vi "Marvin.vi"() -> ()   [LabVIEW 2017]
uses:
  Marvin ATP Remake 1.5.18/PCAN_Driver/ControlCAN.llb/CAN Channel.ctl
  Marvin ATP Remake 6.5.18 - Copy/PCAN_Driver/ControlCAN.llb/DevType.ctl
  Marvin ATP Remake 6.5.18/PCAN_Driver/ControlCAN.llb/VCI_INIT_CONFIG.ctl
  Marvin ATP Remake 6.5.18/PCAN_Driver/ControlCAN.llb/InitFlag.ctl
  Marvin ATP Remake 6.5.18/PCAN_Driver/ControlCAN.llb/Fliter.ctl
  Marvin ATP Remake 6.5.18/PCAN_Driver/ControlCAN.llb/Mode.ctl
  <vilib>/Utility/miscctls.llb/LVMinMaxIncTypeDef.ctl
  PCAN_Driver/ControlCAN.llb/VCI_CAN_OBJ.ctl
  PCAN_Driver/ControlCAN.lvlib
panel:
  out "Array 2":dbl[](array[numeric])
  in  "Clear Data Array":bool
  in  "PlayPause Data Array":bool
  out "CAN Data":cluster{"Frame Data":u64, "Frame ID":u32}[](array[cluster]) {"Frame ID" format="%.0x"; "Frame Data" format="%016x"}
  out "Waveform Chart":dbl[](graph)
  in  "Help Button":bool
  in  "Clear Monitor":bool
  out "Array":u64[][](array[numeric]) format="%016x"
  out "Ambient Over temp":bool
  out "Ambient Sensor temp":bool
  out "Ambient Temperature":dbl
  in  "Motor Over Temp":bool
  in  "Speed control":bool
  out "Unit Adress":string
  in  "Serial Send":bool
  in  "Index":u16(ring) items=["1"=1, "2"=2, "3"=3]
  out "read buffer":string
  in  "SetGet":enum16{"Get", "Set"}(ring)
  in  "Function":T1(ring)
  in  "Value":dbl
  in  "Value 1/2":enum16{"1", "2"}(ring)
  out "Msg Count":u32
  in  "Param to Set":u16(ring) items=["EBAY 5F"=95, "AHU 3F"=63, "AHU 2F"=47]
  out "UUT":u8
  out "Horizontal Progress Bar":i32(slide) min=0 max=48 scale=0.0..50.0
  in  "Set Param.":bool
  in  "Serial Monitor":bool caption="Graph Button"
  in  "Serial Com":bool
  in  "VISA resource name":refnum<visa-resource-name>="COM6"
  out "Serial Status":bool
  in  "Graph Button":bool
  in  "Refresh Button":bool
  out "Data Send":u64 format="%016x"
  in  "Motor Speed RPM":u16
  out "Under voltage/Over voltage":bool
  out "Speed error":bool
  out "Derated drive temp":bool
  out "Motor Over temperature":bool
  out "Commutation err":bool
  out "Motor Sensor temp Fauilre":bool
  out "Drive Over temperature":bool
  out "Drive Sensor temp Failure":bool
  out "Motor Phase Current RMS":dbl
  out "ECS State":u16
  out "Motor Speed RPM":dbl
  out "Motor Stator Temp.":dbl
  out "Power transistor Heat sink Temp.":dbl
  out "DC Current":dbl
  out "DC Voltage":dbl
  in  "Can Send":bool
  in  "Stop":bool
  out "Config_CANAT":T8 {"DevType" items=["USB-CAN"=3, "USB-CAN2"=4]; "CanIndex" items=["通道1", "通道2"]; "VCI_INIT_CONFIG"."Fliter" items=["接收所有类型"=3, "只接收标准帧"=4, "只接收扩展帧"=7]; "VCI_INIT_CONFIG"."Mode" items=["正常工作", "自测模式（环回）", "仅侦听模式"]; "VCI_INIT_CONFIG"."InitFlag" items=["使用Flash参数", "使用界面设置参数"]}
  in  "Channel 2":T3 caption="Channel" items=["Channel 1", "Channel 2"]
  out "CAN Status":bool
  out "Driver Version":string
  out "Hall Sensor Fault":bool
  out "Motor Phase Current":dbl
  in  "Motor Phase Current":u16
  # "ver 1.7c"
  # "Marvin"
  # "REDLER TECHNOLOGIES LTD"
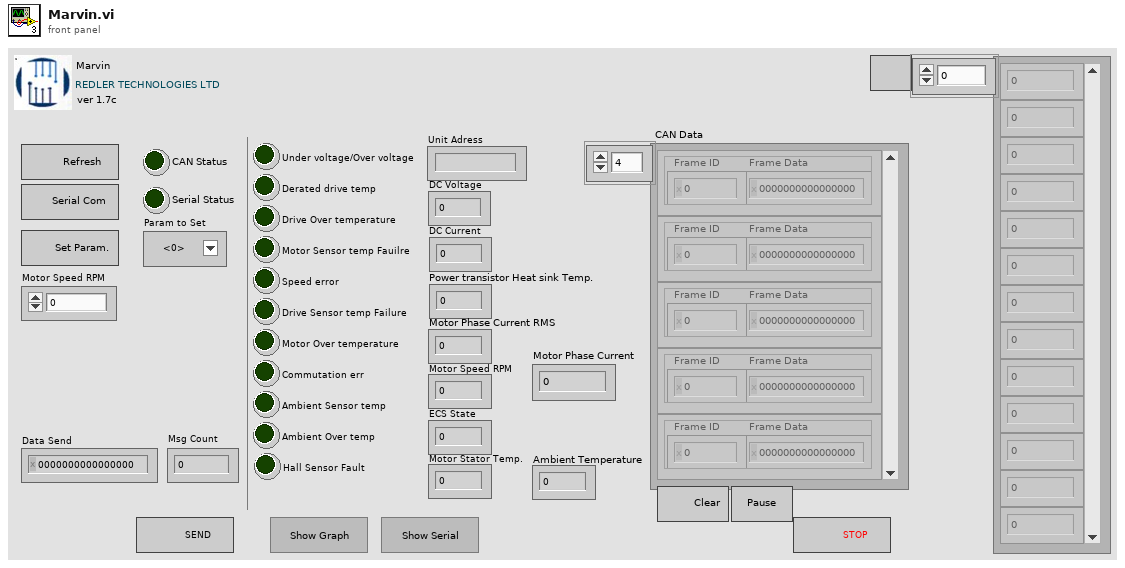
[diagram p1: front panel]
types:
  T1 = enum16{"Enable Conf. EP=1", "Serial Number", "Temperature", "Unit Adress", "Calibration", "Velocity", "Version"}
  T2 = typedef "ControlCAN.lvlib/DevType.ctl" = u32
  T3 = typedef "ControlCAN.lvlib/CAN Channel.ctl" = u32
  T4 = typedef "ControlCAN.lvlib/VCI_INIT_CONFIG.ctl" = cluster{"AccCode":u32, "AccMask":u32, "InitFlag":T5, "Fliter":T6, "Timing0":u8, "Timing1":u8, "Mode":T7}
  T5 = typedef "ControlCAN.lvlib/InitFlag.ctl" = u32
  T6 = typedef "ControlCAN.lvlib/Fliter.ctl" = u8
  T7 = typedef "ControlCAN.lvlib/Mode.ctl" = u8
  T8 = cluster{"DevType":T2, "DevIndex":u32, "CanIndex":T3, "VCI_INIT_CONFIG":T4}
  T9 = cluster{"ID":u32, "MSGTYPE":u8, "LEN":u8, "aDATA":u8[]}[]
  T10 = cluster{"ID":u32, "MSGTYPE":u8, "LEN":u8, "aDATA":u8[]}
  T11 = enum8{"Enabled", "Disabled", "Disabled and Grayed Out"}
  T12 = typedef "LVMinMaxIncTypeDef.ctl" = cluster{"Minimum":dbl, "Maximum":dbl, "Increment":dbl}
  T13 = enum32{"Invalid", "Standard", "Closed", "Hidden", "Minimized", "Maximized"}
  T14 = typedef "ControlCAN.lvlib/VCI_CAN_OBJ.ctl" = cluster{"ID":u32, "TimeStamp":u32, "TimeFlag":u8, "SendType":u8, "RemoteFlag":u8, "ExternFlag":u8, "DataLen":u8, "Data":u8[], "Reserved":u8[]}
  T15 = cluster{"Type":enum16{"接收", "发送"}, "Channel":T3, "Time":timestamp, "VCI_CAN_OBJ":T14}[]
  T16 = cluster{"Type":enum16{"接收", "发送"}, "Channel":T3, "Time":timestamp, "VCI_CAN_OBJ":T14}
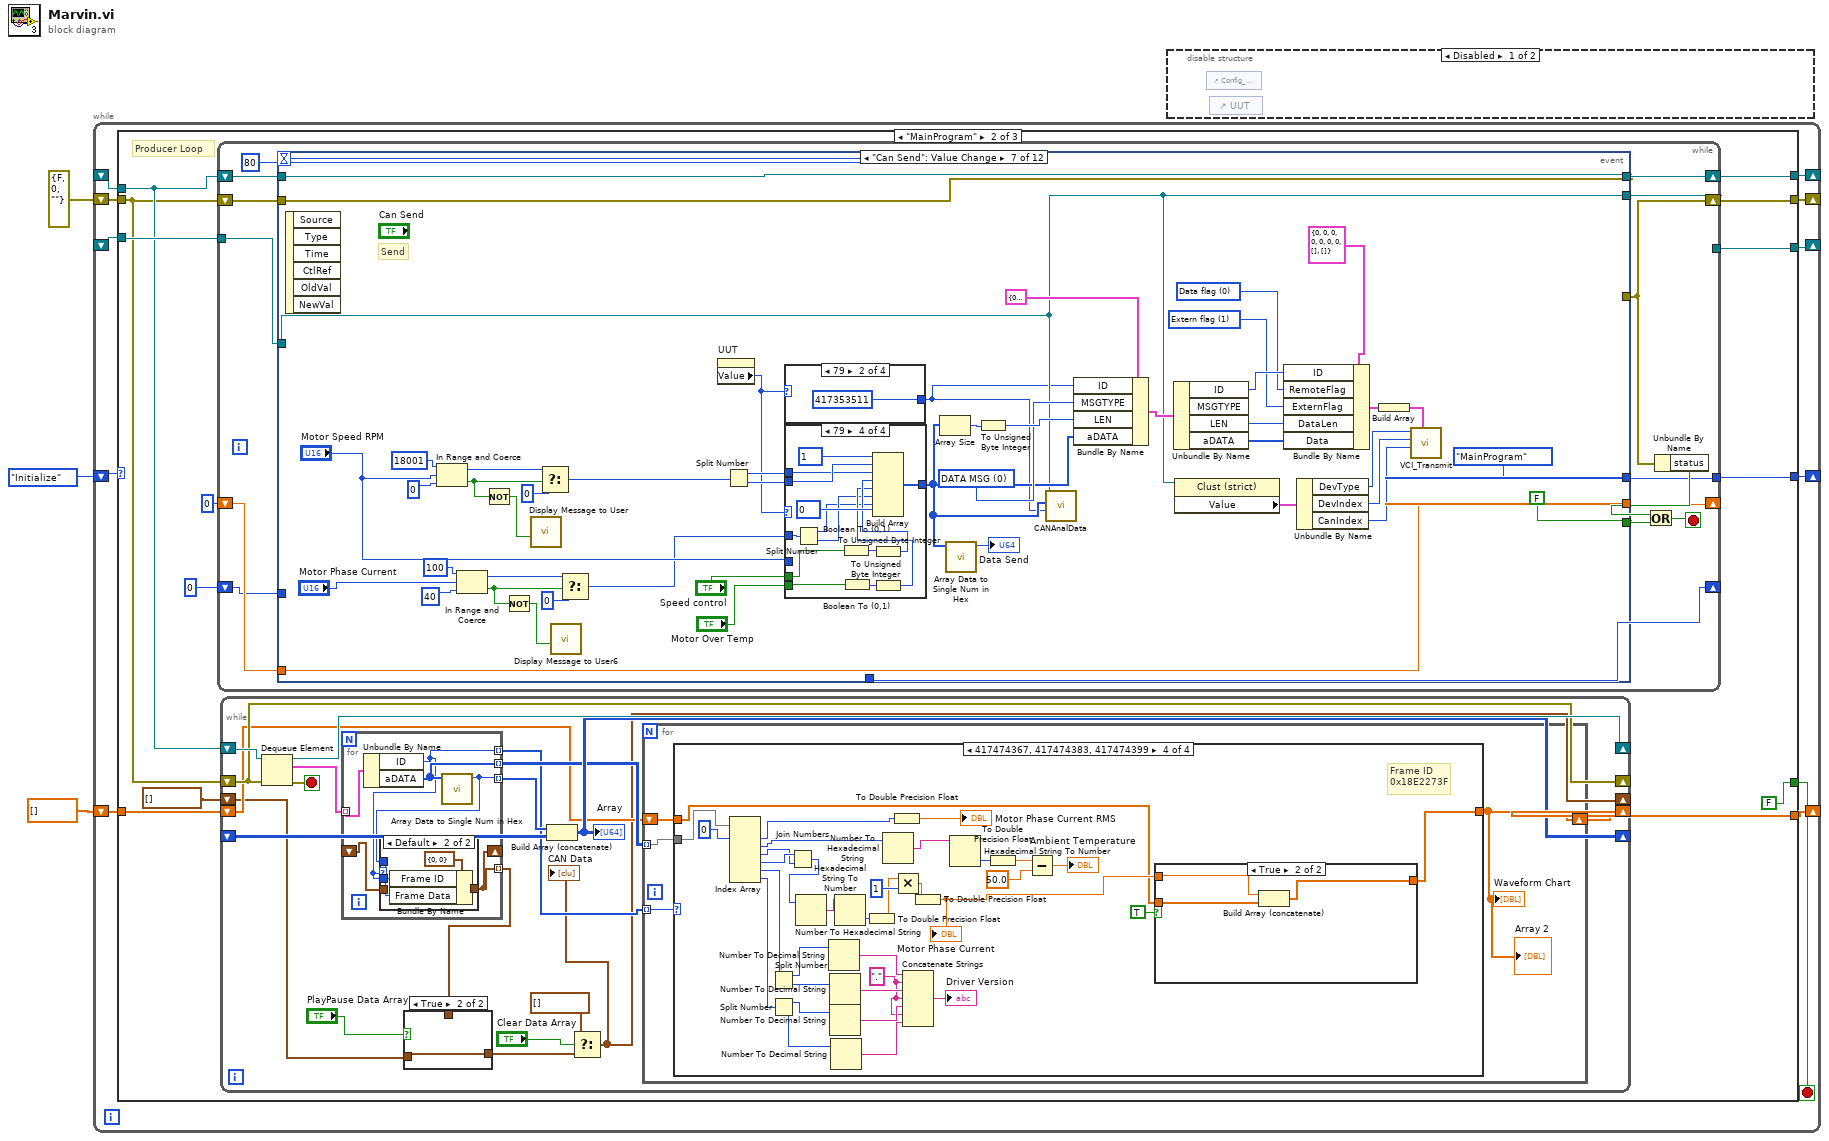
[diagram p0: block diagram]
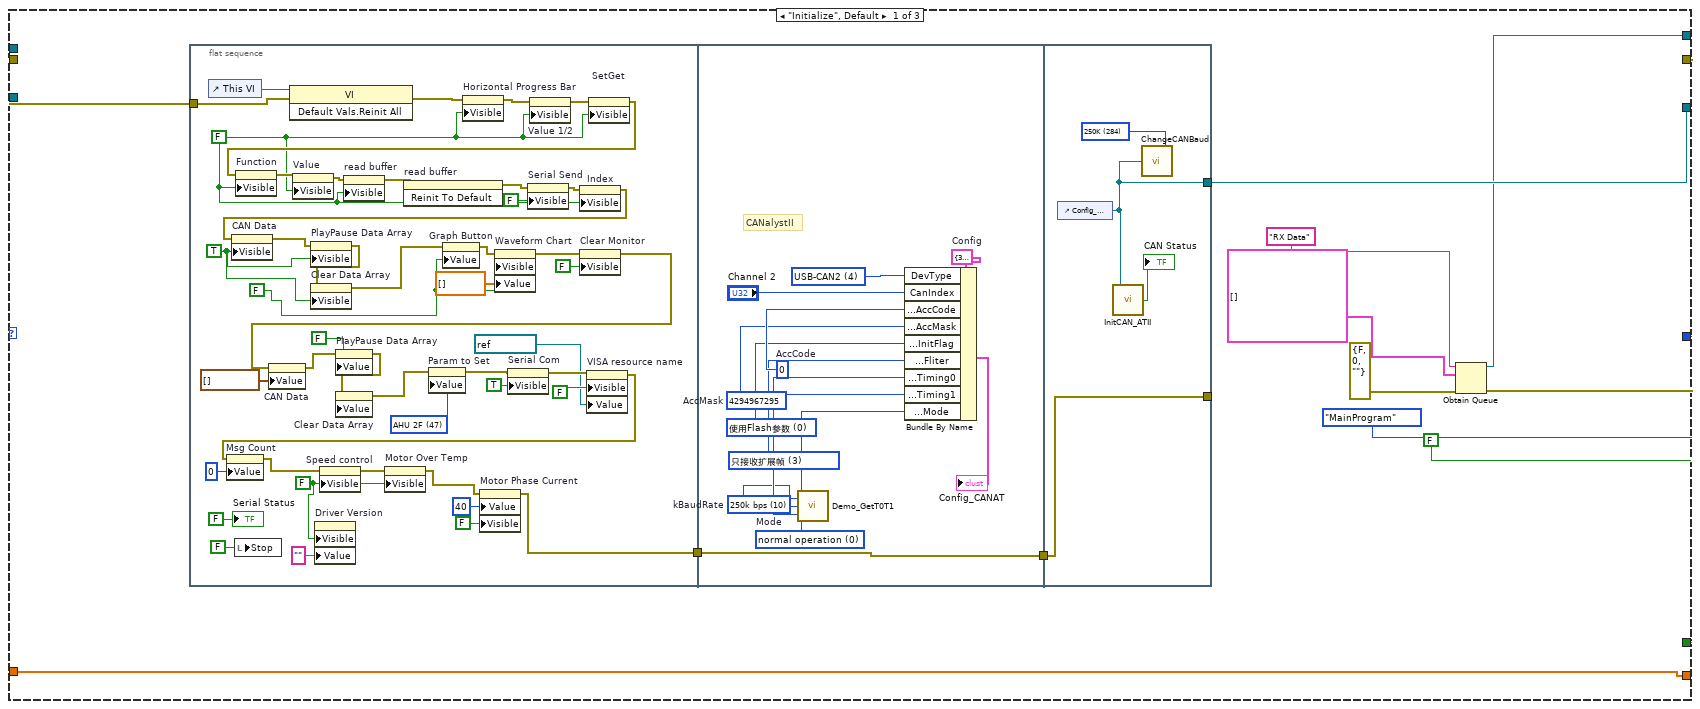
[diagram p3: hidden frame]
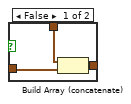
[diagram p4: hidden frame]
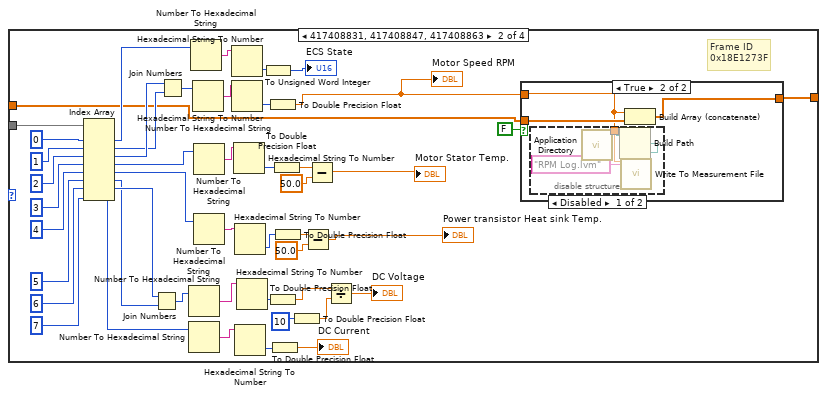
[diagram p6: hidden frame]
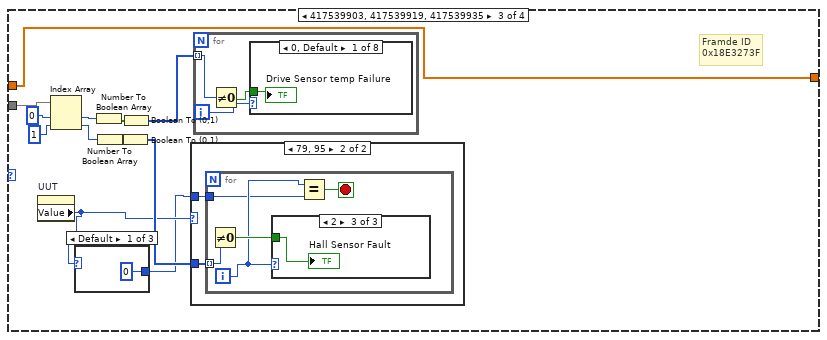
[diagram p9: hidden frame]
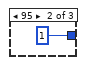
[diagram p10: hidden frame]
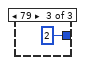
[diagram p11: hidden frame]
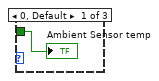
[diagram p13: hidden frame]
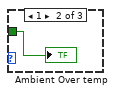
[diagram p14: hidden frame]
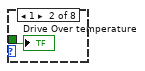
[diagram p15: hidden frame]
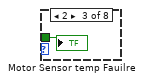
[diagram p16: hidden frame]
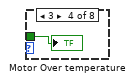
[diagram p17: hidden frame]
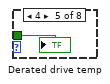
[diagram p18: hidden frame]
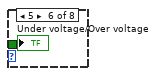
[diagram p19: hidden frame]
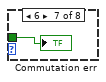
[diagram p20: hidden frame]
diagram:
  n1 = while {
    shift-right: [w9] -> _
    shift-left: enum16{"Stop", "MainProgram", "Initialize"}."Initialize" -> [w14]
    shift-right: [w13] -> _
    shift-left: _ -> [w12]
    shift-right: [w11] -> _
    shift-left: _ -> [w8]
    shift-right: [w10] -> _
    shift-left: errorcluster {"status"=FALSE, "code"=0, "source"=""} ("error out") -> [w7]
    shift-right: [w4] -> _
    shift-left: dbl[] [] -> [w5]
    stop <- w6 stop-if-true
    n2 = case shown="\"MainProgram\"" w14 {
      tunnel: [w26 w100 w1007] -> w13
      tunnel: w12 -> [_ w103 w1007]
      tunnel: [w22 w102 w1008] -> w11
      tunnel: [w21 w101 w1009] -> w10
      tunnel: [enum16{"Stop", "MainProgram", "Initialize"}."MainProgram" w99 enum16{"Stop", "MainProgram", "Initialize"}."Stop"] -> w9
      tunnel: w8 -> [_ w98 w1008]
      tunnel: w7 -> [w19 w97 w1010]
      tunnel: [FALSE ("Stop") FALSE ("Stop") w1006] -> w6
      tunnel: w5 -> [w15 w94 w1004]
      tunnel: [w15 w93 w1004] -> w4
      frame "Initialize", Default {
        n3 = flat-sequence {
          tunnel: w19 -> [w55]
          tunnel: [w29] -> w17
          tunnel: [w74] -> w18
          tunnel: w17 -> [w74]
          tunnel: [w88] -> w26
          tunnel: w18 -> [w87]
          tunnel: [w87] -> _
          frame #0 {
            w38 = FALSE ("PlayPause Data Array")
            w32 = FALSE ("Visible")
            w65 = u16 47 items=["EBAY 5F"=95, "AHU 3F"=63, "AHU 2F"=47] ("Param to Set")
            w33 = TRUE ("Visible")
            w49 = FALSE ("Visible")
            w37 = FALSE ("Graph Button")
            n4 = control-ref of="This VI"() -> (w73:refnum<vi>)
            n5 = local write "Stop"(FALSE ("Stop")) -> ()
            n6 = invoke class="VI" method="Default Vals.Reinit All"(reference=w73, error in=w55) -> (error out=w54:errorcluster)  [unwired: 1 in, 2 out]
            n7 = property on="Driver Version" class="Str"("Visible"=w32, "Value"="" ("Driver Version")) -> ()  [unwired: 2 in, 2 out]
            n8 = property on="Horizontal Progress Bar" class="Slide (strict)"(error in=w54, "Visible"=w49) -> (error out=w63:errorcluster)  [unwired: 1 in, 1 out]
            n9 = property on="Value 1/2" class="Enum (strict)"(error in=w63, "Visible"=w49) -> (error out=w62:errorcluster)  [unwired: 1 in, 1 out]
            n10 = property on="SetGet" class="Enum (strict)"(error in=w62, "Visible"=w49) -> (error out=w61:errorcluster)  [unwired: 1 in, 1 out]
            n11 = property on="Function" class="Enum (strict)"(error in=w61, "Visible"=w49) -> (error out=w60:errorcluster)  [unwired: 1 in, 1 out]
            n12 = property on="Value" class="DigNum (strict)"(error in=w60, "Visible"=w49) -> (error out=w59:errorcluster)  [unwired: 1 in, 1 out]
            n13 = property on="read buffer" class="Str"(error in=w59, "Visible"=w49) -> (error out=w51:errorcluster)  [unwired: 1 in, 1 out]
            n14 = invoke on="read buffer" class="Str" method="Reinit To Default"(error in=w51) -> (error out=w50:errorcluster)  [unwired: 2 in, 2 out]
            n15 = property on="Serial Send" class="Bool (strict)"(error in=w50, "Visible"=FALSE) -> (error out=w58:errorcluster)  [unwired: 1 in, 1 out]
            n16 = property on="Index" class="Ring (strict)"(error in=w58, "Visible"=w49) -> (error out=w44:errorcluster)  [unwired: 1 in, 1 out]
            n17 = property on="CAN Data" class="Arr (strict)"(error in=w44, "Visible"=w33) -> (error out=w36:errorcluster)  [unwired: 1 in, 1 out]
            n18 = property on="PlayPause Data Array" class="Bool (strict)"(error in=w36, "Visible"=w33) -> (error out=w35:errorcluster)  [unwired: 1 in, 1 out]
            n19 = property on="Clear Data Array" class="Bool (strict)"(error in=w35, "Visible"=w33) -> (error out=w34:errorcluster)  [unwired: 1 in, 1 out]
            n20 = property on="Graph Button" class="Bool (strict)"(error in=w34, "Value"=w37) -> (error out=w47:errorcluster)  [unwired: 1 in, 1 out]
            n21 = property on="Waveform Chart" class="WFChart (strict)"(error in=w47, "Visible"=w37, "Value"=dbl[] [] ("Waveform Chart")) -> (error out=w46:errorcluster)  [unwired: 1 in, 1 out]
            n22 = property on="Clear Monitor" class="Bool"(error in=w46, "Visible"=FALSE) -> (error out=w43:errorcluster)  [unwired: 1 in, 1 out]
            n23 = property on="CAN Data" class="Arr (strict)"(error in=w43, "Value"=cluster{"Frame Data":u64, "Frame ID":u32}[] [] ("CAN Data")) -> (error out=w41:errorcluster)  [unwired: 1 in, 1 out]
            n24 = property on="PlayPause Data Array" class="Bool (strict)"(error in=w41, "Value"=w38) -> (error out=w40:errorcluster)  [unwired: 1 in, 1 out]
            n25 = property on="Clear Data Array" class="Bool (strict)"(error in=w40, "Value"=w38) -> (error out=w39:errorcluster)  [unwired: 1 in, 1 out]
            n26 = property on="Param to Set" class="Ring (strict)"(error in=w39, "Value"=w65) -> (error out=w57:errorcluster)  [unwired: 1 in, 1 out]
            n27 = property on="Serial Com" class="Bool"(error in=w57, "Visible"=TRUE) -> (error out=w70:errorcluster)  [unwired: 1 in, 1 out]
            n28 = property on="VISA resource name" class="VISAName"(error in=w70, "Visible"=FALSE, "Value"=refnum<visa-resource-name> "COM1" ("VISA resource name")) -> (error out=w56:errorcluster)  [unwired: 1 in, 1 out]
            n29 = property on="Msg Count" class="DigNum (strict)"(error in=w56, "Value"=u32 0 ("Msg Count")) -> (error out=w53:errorcluster)  [unwired: 1 in, 1 out]
            n30 = property on="Speed control" class="Bool (strict)"(error in=w53, "Visible"=w32) -> (error out=w52:errorcluster)  [unwired: 1 in, 1 out]
            n31 = property on="Motor Over Temp" class="Bool (strict)"(error in=w52, "Visible"=w32) -> (error out=w30:errorcluster)  [unwired: 1 in, 1 out]
            n32 = property on="Motor Phase Current" class="DigNum (strict)"(error in=w30, "Value"=u16 40 ("Motor Phase Current"), "Visible"=FALSE) -> (error out=w29:errorcluster)  [unwired: 1 in, 1 out]
            "Serial Status" <- FALSE ("Serial Status")
          }
          frame #1 {
            w78 = u32 4294967295  # AccMask
            w77 = T5 0 items=["使用Flash参数", "使用界面设置参数"] ("InitFlag")
            w75 = T7 0 items=["normal operation", "Listen-only mode", "test mode"]  # Mode
            w76 = T6 3 items=["接收所有类型"=1, "只接收标准帧"=2, "只接收扩展帧"=3] ("Fliter")
            w82 = u8 10 items=["5k bps"=1, "10k bps"=2, "20k bps"=3, "40k bps"=4, "50k bps"=5, "80k bps"=6, "100k bps"=7, "125k bps"=8, "200k bps"=9, "250k bps"=10, "400k bps"=11, "500k bps"=12, "666k bps"=13, "800k bps"=14, "1000k bps"=15, "33.33k bps"=16, "66.66k bps"=17, "83.33k bps"=18]  # kBaudRate
            w79 = u32 0  # AccCode
            w80 = T2 4 items=["USB-CAN"=3, "USB-CAN2"=4] ("DevType")
            w81 = T8 {"DevType"=3, "DevIndex"=0, "CanIndex"=0, "VCI_INIT_CONFIG"={"AccCode"=0, "AccMask"=0, "InitFlag"=1, "Fliter"=7, "Timing0"=0, "Timing1"=0, "Mode"=0}}  # Config
            # "CANalystII"
            n33 = call "Demo_GetT0T1.vi"("kBaudRate"=w82) -> ("Timing0"=w84:u8, "Timing1"=w85:u8)
            n34 = Bundle By Name(cluster=w81, "DevType"=w80, "CanIndex"="Channel 2", "VCI_INIT_CONFIG.AccCode"=w79, "VCI_INIT_CONFIG.AccMask"=w78, "VCI_INIT_CONFIG.InitFlag"=w77, "VCI_INIT_CONFIG.Fliter"=w76, "VCI_INIT_CONFIG.Timing0"=w84, "VCI_INIT_CONFIG.Timing1"=w85, "VCI_INIT_CONFIG.Mode"=w75) -> (→"Config_CANAT":T8)
          }
          frame #2 {
            w89 = u16 284 items=["1M"=20, "500K"=28, "250K"=284, "125K"=796, "100K"=17199, "50K"=18223, "20K"=21295, "10K"=26415, "5K"=32639] ("baud in")
            n35 = control-ref of="Config_CANAT"() -> (w88:refnum<vi>)
            n36 = call "InitCAN_ATII.vi"("Config"=w88) -> ("Sts"=→"CAN Status":bool)
            n37 = call "ChangeCANBaud.vi"("baud in"=w89, "reference"=w88) -> ()
          }
        }
        n38 = Obtain Queue(name (unnamed)="RX Data", element data type=T9 [], error in (no error)=errorcluster {"status"=FALSE, "code"=0, "source"=""}) -> (queue out=w22:refnum<queue>, error out=w21:errorcluster)  [unwired: 2 in, 1 out]
      }
      frame "MainProgram" {
        # "Producer Loop"
        n39 = while {
          shift-right: [w280] -> w101
          shift-left: w97 -> [w282]
          shift-right: [w281] -> w102
          shift-left: w98 -> [w283]
          tunnel: w103 -> [w284]
          tunnel: [w277] -> w100
          tunnel: [w276] -> w99
          shift-right: [w274] -> _
          shift-left: 0 -> [w275]
          shift-right: [w272] -> _
          shift-left: 0 -> [w273]
          stop <- w285 stop-if-true
          n40 = event shown="[6] \"Can Send\": Value Change" {
            selector: _ -> [_ _ _ _ _ _ _ _ _ _ _ _]
            dyn-events: _ -> [_ _ _ _ _ _ _ _ _ _ _ _]
            timeout: 80 ("Numeric") -> [_ _ _ _ _ _ _ _ _ _ _ _]
            tunnel: w284 -> [w306 w384 w403 w470 w725 w823 w853 w944 w964 w981 w996 w1002]
            tunnel: w283 -> [w303 w385 w406 w471 w724 w824 w874 w945 w963 w982 w993 w999]
            tunnel: w282 -> [w288 w383 w401 w458 w717 w816 w873 w924 w959 w974 w992 w1000]
            tunnel: [w301 w385 w406 w471 w724 w824 w874 w945 w963 w982 w991 w999] -> w281
            tunnel: [w300 w378 w402 w463 w713 w813 w873 w931 w956 w972 w989 w998] -> w280
            tunnel: [FALSE ("Stop") FALSE ("Stop") FALSE ("Stop") FALSE ("Stop") FALSE ("Stop") FALSE ("Stop") FALSE ("Stop") FALSE ("Stop") FALSE ("Stop") FALSE ("Stop") TRUE ("Stop") TRUE ("Stop")] -> w278
            tunnel: [w299 w384 w403 w470 w725 w823 w853 w944 w964 w981 w996 w1002] -> w277
            tunnel: [enum16{"Stop", "MainProgram", "Initialize"}."MainProgram" enum16{"Stop", "MainProgram", "Initialize"}."MainProgram" enum16{"Stop", "MainProgram", "Initialize"}."MainProgram" enum16{"Stop", "MainProgram", "Initialize"}."MainProgram" enum16{"Stop", "MainProgram", "Initialize"}."MainProgram" enum16{"Stop", "MainProgram", "Initialize"}."MainProgram" enum16{"Stop", "MainProgram", "Initialize"}."MainProgram" enum16{"Stop", "MainProgram", "Initialize"}."MainProgram" enum16{"Stop", "MainProgram", "Initialize"}."MainProgram" enum16{"Stop", "MainProgram", "Initialize"}."MainProgram" enum16{"Stop", "MainProgram", "Initialize"}."Stop" enum16{"Stop", "MainProgram", "Initialize"}."Initialize"] -> w276
            tunnel: w275 -> [w295 w388 w399 w459 w715 w827 w839 w940 w955 w970 w988 w997]
            tunnel: [w294 w388 w399 w459 w715 w827 w839 w940 w955 w970 w988 w997] -> w274
            tunnel: w273 -> [w287 _ _ _ _ _ _ _ _ _ _ _]
            tunnel: [w287 _ _ _ _ _ _ _ _ _ _ _] -> w272
            event Timeout {
              n41 = event-data() -> ()  [unwired: 1 in, 3 out]
              n42 = property class="Clust (strict)"(reference=w306) -> (reference out=w299:refnum<vi>, "Value"=w307:T8)  [unwired: 1 in, 1 out]
              n43 = property on="Speed control" class="Bool (strict)"(error in=w288) -> ("Value"=w289:bool)  [unwired: 1 in, 2 out]
              n44 = case shown="True" w289 {
                frame False {
                }
                frame True {
                  n45 = property on="Motor Speed RPM" class="DigNum (strict)"() -> ("Value"=w313:u16)  [unwired: 2 in, 2 out]
                  n46 = control-ref of="Config_CANAT"() -> (w312:refnum<vi>)
                  n47 = control-ref of="UUT"() -> (w311:refnum<vi>)
                  n48 = call "CANSendMotorSpeed.vi"("Remote"=TRUE, "Motor Speed RPM"=w313, "UUT"=w311, "CAN Cluster in"=w312) -> ()  [unwired: 7 in, 1 out]
                }
              }
              n49 = Unbundle By Name(w307) -> ("DevType"=w308:T2, "CanIndex"=w304:T3)
              n50 = property on="Horizontal Progress Bar" class="Slide (strict)"(error in=w288, "Visible"=FALSE) -> (error out=w290:errorcluster)  [unwired: 1 in, 1 out]
              n51 = call "VCI_Receive.vi"("CANIndex"=w304, "DevIndex"=u32 0, "DevType"=w308) -> ("Recieve"=w302:T14[])  [unwired: 3 in, 5 out]
              n52 = Empty Array?(array=w302) -> (empty?=w305:bool)
              n53 = case shown="False" w305 {
                tunnel: w304 -> [w325 _]
                tunnel: w299 -> [w323 _]
                tunnel: w303 -> [w322 w377]
                tunnel: w290 -> [w321 w376]
                tunnel: w302 -> [w326 _]
                tunnel: [w316 w376] -> w300
                tunnel: [w315 w377] -> w301
                tunnel: [w314 0] -> w291
                frame False {
                  n54 = call "Demo_MakeDispBuff.vi"("Channel"=w325, "Type"=enum16{"接收", "发送"}."接收", "OBJs"=w326) -> ("Buffer"=w324:T15)
                  n55 = for {
                    N: 3 -> [_]
                    tunnel: w324 -> [w340]
                    tunnel: w323 -> [w339]
                    tunnel: w322 -> [w330]
                    tunnel: w321 -> [w329]
                    tunnel: [w332] -> w319 mode=indexing
                    tunnel: [w330] -> w318
                    tunnel: [w329] -> w317
                    tunnel: [w328] -> w314
                    i -> [w328]
                    n56 = property class="Clust (strict)"(reference=w339) -> ("Value"=w337:T8)  [unwired: 1 in, 2 out]
                    n57 = Index Array(array=w340, index=w328) -> (element=w333:T16)
                    n58 = Unbundle By Name(w333) -> ("Channel"=w335:T3, "VCI_CAN_OBJ"=w338:T14)  [unwired: 2 out]
                    n59 = Unbundle By Name(w337) -> ("CanIndex"=w336:T3)
                    n60 = Equal?(x=w336, y=w335) -> (x = y?=w334:bool)
                    n61 = case shown="True" w334 {
                      tunnel: w338 -> [_ w356]
                      tunnel: [w341 w352] -> w332
                      tunnel: T10 {"ID"=0, "MSGTYPE"=0, "LEN"=0, "aDATA"=[]} ("Msg") -> [w341 w351]
                      frame False {
                      }
                      frame True {
                        n62 = Unbundle By Name(w356) -> ("ID"=w350:u32, "DataLen"=w355:u8, "Data"=w353:u8[])
                        n63 = Bundle By Name(cluster=w351, "ID"=w350, "MSGTYPE"=u8 0, "LEN"=w355, "aDATA"=w353) -> (w352:T10)
                        n64 = Unbundle By Name(w352) -> ("ID"=w348:u32)
                        n65 = Split Number(x=w348) -> (lo(x)=w349:u16)  [unwired: 1 out]
                        n66 = Split Number(x=w349) -> (lo(x)=w346:u8)  [unwired: 1 out]
                        "UUT" <- w346
                        n67 = case shown="95" w346 {
                          tunnel: ["EBAY 5F" "PUMP 4F" w369 "AHU 3F" "AHU 2F"] -> w345
                          tunnel: [TRUE w366 w370 w371 w373] -> w343
                          tunnel: [TRUE w366 w368 w371 w373] -> w342
                          frame 95 {
                          }
                          frame 79 {
                            w366 = TRUE
                          }
                          frame Default {
                            n68 = property on="Hall Sensor Fault" class="Bool (strict)"() -> ("Visible"=w368:bool)  [unwired: 2 in, 2 out]
                            n69 = property on="Speed control" class="Bool (strict)"() -> ("Visible"=w370:bool)  [unwired: 2 in, 2 out]
                            n70 = property on="Unit Adress" class="Str"() -> ("Value"=w369:string)  [unwired: 2 in, 2 out]
                          }
                          frame 63 {
                            w371 = FALSE
                          }
                          frame 47 {
                            w373 = FALSE
                          }
                        }
                        n71 = Not Equal To 0?(x=w346) -> (x != 0?=w347:bool)
                        n72 = case shown="True" w347 {
                          tunnel: w346 -> [_ w362]
                          tunnel: w345 -> [_ w359]
                          tunnel: [w357 w358] -> w344
                          frame False {
                            n73 = property on="Unit Adress" class="Str"() -> ("Value"=w357:string)  [unwired: 2 in, 2 out]
                          }
                          frame True {
                            n74 = Number To Decimal String(number=w362) -> (decimal integer string=w361:string)  [unwired: 1 in]
                            n75 = call <vilib>:"Space Constant.vi"() -> ("String"=w360:string)
                            n76 = Concatenate Strings(w361, w360, w359) -> (w358:string)
                          }
                        }
                        "Unit Adress" <- w344
                        n77 = property on="Driver Version" class="Str"("Visible"=w343) -> ()  [unwired: 2 in, 2 out]
                        n78 = property on="Hall Sensor Fault" class="Bool (strict)"("Visible"=w342) -> ()  [unwired: 2 in, 2 out]
                        n79 = property on="Motor Phase Current" class="DigNum (strict)"("Visible"=w342) -> ()  [unwired: 2 in, 2 out]
                        n80 = property on="Motor Phase Current" class="DigNum (strict)"("Visible"=w342) -> ()  [unwired: 2 in, 2 out]
                        n81 = property on="Ambient Over temp" class="Bool (strict)"("Visible"=w343) -> ()  [unwired: 2 in, 2 out]
                        n82 = property on="Ambient Sensor temp" class="Bool (strict)"("Visible"=w343) -> ()  [unwired: 2 in, 2 out]
                        n83 = property on="Ambient Temperature" class="DigNum (strict)"("Visible"=w343) -> ()  [unwired: 2 in, 2 out]
                        n84 = property on="Motor Over Temp" class="Bool (strict)"("Visible"=w343) -> ()  [unwired: 2 in, 2 out]
                        n85 = property on="Speed control" class="Bool (strict)"("Visible"=w343) -> ()  [unwired: 2 in, 2 out]
                      }
                    }
                  }
                  n86 = Enqueue Element(queue=w318, element=w319, error in (no error)=w317) -> (queue out=w315:refnum<queue>, error out=w316:errorcluster)  [unwired: 2 out]
                }
                frame True {
                }
              }
              n87 = Divide(x=w291, y=u32 2) -> (x/y=w292:dbl)
              n88 = Add(x=w292, y=w295) -> (x+y=w294:dbl)
              "Msg Count" <- w294
            }
            event "Clear Monitor": Value Change {
              n89 = event-data() -> ()  [unwired: 1 in, 6 out]
              n90 = property on="VISA resource name" class="VISAName"(error in=w383) -> (error out=w382:errorcluster, "Value"=w381:refnum<visa-resource-name>)  [unwired: 1 in, 1 out]
              n91 = disable-structure shown="Enabled" {
                disable-tunnel: w382 -> [w393 w396]
                disable-tunnel: w381 -> [w391 w397]
                disable-tunnel: [w390 ""] -> w380
                disable-tunnel: [w389 w395] -> w379
                frame Disabled {
                  n92 = call "Serial.vi"("error in (no error)"=w393, "Clear Log"=TRUE, "VISA resource name"=w391) -> ("error out"=w389:errorcluster, "read buffer"=w390:string)  [unwired: 7 in]
                }
                frame Enabled {
                  n93 = VISA Flush I/O Buffer(VISA resource name=w397, error in (no error)=w396) -> (error out=w395:errorcluster)  [unwired: 1 in, 1 out]
                }
              }
              n94 = property on="read buffer" class="Str"(error in=w379, "Value"=w380) -> (error out=w378:errorcluster)  [unwired: 1 in, 1 out]
            }
            event "Serial Monitor": Value Change {
              n95 = event-data() -> ()  [unwired: 1 in, 6 out]
              n96 = property on="Serial Status" class="Bool (strict)"(error in=w401) -> (error out=w400:errorcluster, "Value"=w398:bool)  [unwired: 1 in, 1 out]
              n97 = case shown="True" w398 {
                tunnel: w400 -> [w410 w423]
                tunnel: [w408 w428] -> w402
                frame False {
                  n98 = call "Display Message to User3"("error in (no error)"=w410) -> ("error out"=w409:errorcluster)  [unwired: 9 in, 1 out]
                  n99 = property on="Serial Monitor" class="Bool (strict)"(error in=w409, "Value"=FALSE ("Serial Monitor")) -> (error out=w408:errorcluster)  [unwired: 1 in, 1 out]
                }
                frame True {
                  w415 = FALSE ("Visible")
                  w425 = FALSE ("Visible")
                  w426 = u16 1 items=["1"=1, "2"=2, "3"=3] ("Index")
                  n100 = property on="Index" class="Ring (strict)"(error in=w423, "Value"=w426) -> (error out=w422:errorcluster)  [unwired: 1 in, 1 out]
                  n101 = property on="Value 1/2" class="Enum (strict)"(error in=w422, "Visible"=w425) -> (error out=w421:errorcluster)  [unwired: 1 in, 1 out]
                  n102 = property on="Value" class="DigNum (strict)"(error in=w421, "Visible"=w425) -> (error out=w420:errorcluster)  [unwired: 1 in, 1 out]
                  n103 = property on="SetGet" class="Enum (strict)"(error in=w420, "Value"=enum16{"Get", "Set"}."Get" ("SetGet")) -> (error out=w419:errorcluster)  [unwired: 1 in, 1 out]
                  n104 = property on="Serial Send" class="Bool (strict)"(error in=w419, "Visible"=w415) -> (error out=w414:errorcluster)  [unwired: 1 in, 1 out]
                  n105 = property on="Clear Monitor" class="Bool"(error in=w414, "Visible"=w415) -> (error out=w413:errorcluster)  [unwired: 1 in, 1 out]
                  n106 = property on="Function" class="Enum (strict)"(error in=w413, "Value"=T1."Serial Number" ("Function")) -> (error out=w418:errorcluster)  [unwired: 1 in, 1 out]
                  n107 = property on="Index" class="Ring (strict)"(error in=w418, "DisabledEnum"=T11."Disabled and Grayed Out" ("Disabled")) -> (error out=w416:errorcluster)  [unwired: 1 in, 1 out]
                  n108 = case shown="True" "Serial Monitor" {
                    selector: "Serial Monitor" -> [w432 w453]
                    tunnel: w416 -> [w431 w449]
                    tunnel: [w434 w450] -> w428
                    tunnel: [FALSE TRUE] -> w412
                    frame False {
                      n109 = property on="Graph Button" class="Bool (strict)"(error in=w431) -> (error out=w430:errorcluster, "Value"=w429:bool)  [unwired: 1 in, 1 out]
                      n110 = case shown="True" w429 {
                        tunnel: [w438 w443] -> w435
                        tunnel: w430 -> [w440 w446]
                        tunnel: w432 -> [w441 _]
                        frame False {
                          n111 = property on="Waveform Chart" class="WFChart (strict)"(error in=w440, "Visible"=FALSE) -> (error out=w437:errorcluster)  [unwired: 1 in, 1 out]
                          n112 = Not(x=w441) -> (.not. x?=w436:bool)
                          n113 = property on="PlayPause Data Array" class="Bool (strict)"("Visible"=w436) -> ()  [unwired: 2 in, 2 out]
                          n114 = property on="Clear Data Array" class="Bool (strict)"("Visible"=w436) -> ()  [unwired: 2 in, 2 out]
                          n115 = property on="CAN Data" class="Arr (strict)"(error in=w437, "Visible"=w436) -> (error out=w438:errorcluster)  [unwired: 1 in, 1 out]
                        }
                        frame True {
                          w442 = FALSE ("Visible")
                          n116 = property on="Waveform Chart" class="WFChart (strict)"(error in=w446, "Visible"=TRUE) -> (error out=w444:errorcluster)  [unwired: 1 in, 1 out]
                          n117 = property on="PlayPause Data Array" class="Bool (strict)"("Visible"=w442) -> ()  [unwired: 2 in, 2 out]
                          n118 = property on="Clear Data Array" class="Bool (strict)"("Visible"=w442) -> ()  [unwired: 2 in, 2 out]
                          n119 = property on="CAN Data" class="Arr (strict)"(error in=w444, "Visible"=w442) -> (error out=w443:errorcluster)  [unwired: 1 in, 1 out]
                        }
                      }
                      n120 = property on="Serial Monitor" class="Bool (strict)"(error in=w435, "Value"=w432) -> (error out=w434:errorcluster)  [unwired: 1 in, 1 out]
                    }
                    frame True {
                      n121 = Not(x=w453) -> (.not. x?=w447:bool)
                      n122 = property on="PlayPause Data Array" class="Bool (strict)"("Visible"=w447) -> ()  [unwired: 2 in, 2 out]
                      n123 = property on="CAN Data" class="Arr (strict)"(error in=w449, "Visible"=w447) -> (error out=w448:errorcluster)  [unwired: 1 in, 1 out]
                      n124 = property on="Clear Data Array" class="Bool (strict)"("Visible"=w447) -> ()  [unwired: 2 in, 2 out]
                      n125 = property on="Serial Monitor" class="Bool (strict)"(error in=w448, "Value"=w453) -> (error out=w452:errorcluster)  [unwired: 1 in, 1 out]
                      n126 = property on="Graph Button" class="Bool (strict)"(error in=w452, "Value"=w447) -> (error out=w451:errorcluster)  [unwired: 1 in, 1 out]
                      n127 = property on="Waveform Chart" class="WFChart (strict)"(error in=w451, "Visible"=w447) -> (error out=w450:errorcluster)  [unwired: 1 in, 1 out]
                    }
                  }
                  n128 = property on="SetGet" class="Enum (strict)"("Visible"=w412) -> ()  [unwired: 2 in, 2 out]
                  n129 = property on="Index" class="Ring (strict)"("Visible"=w412) -> ()  [unwired: 2 in, 2 out]
                  n130 = property on="Function" class="Enum (strict)"("Visible"=w412) -> ()  [unwired: 2 in, 2 out]
                  n131 = property on="Clear Monitor" class="Bool"("Visible"=w412) -> ()  [unwired: 2 in, 2 out]
                  n132 = property on="Serial Send" class="Bool (strict)"("Visible"=w412) -> ()  [unwired: 2 in, 2 out]
                  n133 = property on="read buffer" class="Str"("Visible"=w412) -> ()  [unwired: 2 in, 2 out]
                }
              }
            }
            event "Serial Send", "Function", "SetGet": Value Change {
              n134 = event-data() -> ()  [unwired: 1 in, 6 out]
              n135 = case shown="\"Enable Conf. EP=1\"" "Function" {
                tunnel: w458 -> [w477 w482 w489 w491 w494 w498 w500 w501]
                tunnel: [w476 w484 w488 w493 w496 w497 w500 w501] -> w456
                frame "Serial Number" {
                  n136 = property on="Index" class="Ring (strict)"(error in=w477, "DisabledEnum"=T11."Disabled and Grayed Out" ("Disabled")) -> (error out=w476:errorcluster)  [unwired: 1 in, 1 out]
                }
                frame "Temperature" {
                  n137 = property on="UUT" class="DigNum (strict)"() -> ("Value"=w479:u8)  [unwired: 2 in, 2 out]
                  n138 = case shown="95" w479 {
                    tunnel: [i32[] [2] ("Disabled Items []") i32[] [3] ("Disabled Items []")] -> w480
                    frame 47, 63, Default {
                    }
                    frame 95 {
                    }
                  }
                  n139 = property on="Index" class="Ring (strict)"(error in=w482, "DisabledEnum"=T11."Enabled" ("Disabled"), "Visible"=TRUE, "Disabled Items []"=w480) -> (error out=w484:errorcluster)  [unwired: 1 in, 1 out]
                }
                frame "Unit Adress" {
                  n140 = property on="Index" class="Ring (strict)"(error in=w489, "DisabledEnum"=T11."Enabled" ("Disabled"), "Visible"=TRUE) -> (error out=w488:errorcluster)  [unwired: 1 in, 1 out]
                }
                frame "Calibration" {
                  n141 = property on="Index" class="Ring (strict)"(error in=w491, "DisabledEnum"=T11."Disabled and Grayed Out" ("Disabled")) -> (error out=w493:errorcluster)  [unwired: 1 in, 1 out]
                }
                frame "Velocity" {
                  n142 = property on="Index" class="Ring (strict)"(error in=w494, "DisabledEnum"=T11."Disabled and Grayed Out" ("Disabled")) -> (error out=w496:errorcluster)  [unwired: 1 in, 1 out]
                }
                frame "Version" {
                  n143 = property on="Index" class="Ring (strict)"(error in=w498, "DisabledEnum"=T11."Disabled and Grayed Out" ("Disabled")) -> (error out=w497:errorcluster)  [unwired: 1 in, 1 out]
                }
                frame "Enable Conf. EP=1" {
                }
                frame Default {
                }
              }
              n144 = property on="VISA resource name" class="VISAName"() -> ("Value"=w472:refnum<visa-resource-name>)  [unwired: 2 in, 2 out]
              n145 = property on="read buffer" class="Str"(error in=w456) -> (error out=w465:errorcluster, "Text.Scroll Position"=w462:u32)  [unwired: 1 in, 1 out]
              n146 = case shown="\"Set\"" "SetGet" {
                tunnel: "Function" -> [w505 w604]
                tunnel: w472 -> [w511 w614]
                tunnel: w465 -> [w508 w603]
                tunnel: "Value" -> [_ w613]
                tunnel: "Value 1/2" -> [_ w611]
                tunnel: "Index" -> [w506 w608]
                tunnel: [w510 w606] -> w464
                tunnel: [w503 w605] -> w469
                tunnel: "Serial Send" -> [w502 w595]
                frame "Get", Default {
                  w509 = FALSE ("Visible")
                  n147 = property on="Value" class="DigNum (strict)"(error in=w508, "Visible"=w509) -> (error out=w507:errorcluster)  [unwired: 1 in, 1 out]
                  n148 = property on="Value 1/2" class="Enum (strict)"(error in=w507, "Visible"=w509) -> (error out=w504:errorcluster)  [unwired: 1 in, 1 out]
                  n149 = case shown="True" w502 {
                    tunnel: w511 -> [_ w522]
                    tunnel: [w512 w517] -> w510
                    tunnel: w506 -> [_ w521]
                    tunnel: w505 -> [_ w520]
                    tunnel: w504 -> [w512 w519]
                    tunnel: [w513 w515] -> w503
                    frame False {
                      n150 = property on="read buffer" class="Str"() -> ("Value"=w513:string)  [unwired: 2 in, 2 out]
                    }
                    frame True {
                      n151 = case shown="\"Serial Number\"" w520 {
                        tunnel: w522 -> [w527 w545 w561 w570 w577 w588 _]
                        tunnel: w519 -> [w525 w536 w551 w565 w575 w586 w593]
                        tunnel: [w530 w546 w562 w571 w581 w589 w593] -> w517
                        tunnel: [w529 w547 w560 w572 w582 w584 "Cannot perform operation.\n" ("read buffer")] -> w516
                        tunnel: w521 -> [_ w540 w553 _ _ _ _]
                        frame "Serial Number" {
                          n152 = property on="Index" class="Ring (strict)"(error in=w525, "DisabledEnum"=T11."Disabled and Grayed Out" ("Disabled")) -> (error out=w524:errorcluster)  [unwired: 1 in, 1 out]
                          n153 = Concatenate Strings("SN" ("string"), "\r\n" ("write buffer")) -> (w528:string)
                          n154 = call "Serial.vi"("error in (no error)"=w524, "Clear Log"=FALSE, "write buffer"=w528, "VISA resource name"=w527) -> ("error out"=w530:errorcluster, "read buffer"=w529:string)  [unwired: 6 in]
                        }
                        frame "Temperature" {
                          n155 = Number To Decimal String(number=w540) -> (decimal integer string=w539:string)  [unwired: 1 in]
                          n156 = property on="Index" class="Ring (strict)"(error in=w536, "DisabledEnum"=T11."Enabled" ("Disabled"), "Visible"=TRUE) -> (error out=w535:errorcluster)  [unwired: 1 in, 1 out]
                          n157 = Concatenate Strings("TA" ("string"), "[", w539, "]", "\r\n" ("write buffer")) -> (w541:string)
                          n158 = call "Serial.vi"("error in (no error)"=w535, "Clear Log"=FALSE, "write buffer"=w541, "VISA resource name"=w545) -> ("error out"=w546:errorcluster, "read buffer"=w547:string)  [unwired: 6 in]
                        }
                        frame "Unit Adress" {
                          n159 = Number To Decimal String(number=w553) -> (decimal integer string=w559:string)  [unwired: 1 in]
                          n160 = property on="Index" class="Ring (strict)"(error in=w551, "DisabledEnum"=T11."Enabled" ("Disabled"), "Visible"=TRUE) -> (error out=w550:errorcluster)  [unwired: 1 in, 1 out]
                          n161 = Concatenate Strings("UA" ("string"), "[", w559, "]", "\r\n" ("write buffer")) -> (w554:string)
                          n162 = call "Serial.vi"("error in (no error)"=w550, "Clear Log"=FALSE, "write buffer"=w554, "VISA resource name"=w561) -> ("error out"=w562:errorcluster, "read buffer"=w560:string)  [unwired: 6 in]
                        }
                        frame "Calibration" {
                          n163 = property on="Index" class="Ring (strict)"(error in=w565, "DisabledEnum"=T11."Disabled and Grayed Out" ("Disabled")) -> (error out=w564:errorcluster)  [unwired: 1 in, 1 out]
                          n164 = Concatenate Strings("CC" ("string"), "\r\n" ("write buffer")) -> (w568:string)
                          n165 = call "Serial.vi"("error in (no error)"=w564, "Clear Log"=FALSE, "write buffer"=w568, "VISA resource name"=w570) -> ("error out"=w571:errorcluster, "read buffer"=w572:string)  [unwired: 6 in]
                        }
                        frame "Velocity" {
                          n166 = property on="Index" class="Ring (strict)"(error in=w575, "DisabledEnum"=T11."Disabled and Grayed Out" ("Disabled")) -> (error out=w574:errorcluster)  [unwired: 1 in, 1 out]
                          n167 = Concatenate Strings("VC" ("string"), "\r\n" ("write buffer")) -> (w578:string)
                          n168 = call "Serial.vi"("error in (no error)"=w574, "Clear Log"=FALSE, "write buffer"=w578, "VISA resource name"=w577) -> ("error out"=w581:errorcluster, "read buffer"=w582:string)  [unwired: 6 in]
                        }
                        frame "Version" {
                          n169 = Concatenate Strings("VR" ("string"), "\r\n" ("write buffer")) -> (w590:string)
                          n170 = property on="Index" class="Ring (strict)"(error in=w586, "DisabledEnum"=T11."Disabled and Grayed Out" ("Disabled")) -> (error out=w585:errorcluster)  [unwired: 1 in, 1 out]
                          n171 = call "Serial.vi"("error in (no error)"=w585, "Clear Log"=FALSE, "write buffer"=w590, "VISA resource name"=w588) -> ("error out"=w589:errorcluster, "read buffer"=w584:string)  [unwired: 6 in]
                        }
                        frame Default {
                        }
                      }
                      n172 = property on="Serial Send" class="Bool (strict)"(error in=w517, "Value"=FALSE ("Serial Send")) -> ()  [unwired: 1 in, 2 out]
                      n173 = property on="read buffer" class="Str"() -> ("Value"=w514:string)  [unwired: 2 in, 2 out]
                      n174 = Concatenate Strings(w514, w516) -> (w515:string)
                    }
                  }
                }
                frame "Set" {
                  n175 = To Unsigned Long Integer(number=w613) -> (unsigned 32bit integer=w609:u32)
                  n176 = Number To Decimal String(number=w608) -> (decimal integer string=w607:string)  [unwired: 1 in]
                  n177 = Number To Decimal String(number=w611) -> (decimal integer string=w610:string)  [unwired: 1 in]
                  n178 = case shown="Default" w604 {
                    tunnel: w603 -> [w688 w692 w696 w700 w704 w708 w710 w712]
                    tunnel: [FALSE TRUE TRUE FALSE FALSE FALSE w709 w711] -> w601
                    tunnel: [TRUE TRUE TRUE FALSE TRUE FALSE w709 w711] -> w600
                    tunnel: [FALSE FALSE FALSE TRUE FALSE FALSE w709 w711] -> w599
                    tunnel: [w688 w692 w696 w700 w704 w708 w710 w712] -> w597
                    frame "Serial Number" {
                    }
                    frame "Temperature" {
                    }
                    frame "Unit Adress" {
                    }
                    frame "Calibration" {
                    }
                    frame "Velocity" {
                    }
                    frame "Version" {
                    }
                    frame "Enable Conf. EP=1" {
                      w709 = FALSE
                    }
                    frame Default {
                      w711 = FALSE
                    }
                  }
                  n179 = Number To Decimal String(number=w609) -> (decimal integer string=w612:string)  [unwired: 1 in]
                  n180 = property on="Index" class="Ring (strict)"(error in=w597, "Visible"=w601) -> (error out=w602:errorcluster)  [unwired: 1 in, 1 out]
                  n181 = property on="Value" class="DigNum (strict)"(error in=w602, "Visible"=w600) -> (error out=w598:errorcluster)  [unwired: 1 in, 1 out]
                  n182 = property on="Value 1/2" class="Enum (strict)"(error in=w598, "Visible"=w599) -> (error out=w596:errorcluster)  [unwired: 1 in, 1 out]
                  n183 = case shown="True" w595 {
                    tunnel: w614 -> [_ w628]
                    tunnel: w612 -> [_ w627]
                    tunnel: w610 -> [_ w626]
                    tunnel: w609 -> [_ w625]
                    tunnel: w607 -> [_ w624]
                    tunnel: [w615 w623] -> w606
                    tunnel: [w616 w622] -> w605
                    tunnel: w604 -> [_ w620]
                    tunnel: w596 -> [w615 w619]
                    frame False {
                      n184 = property on="read buffer" class="Str"() -> ("Value"=w616:string)  [unwired: 2 in, 2 out]
                    }
                    frame True {
                      n185 = flat-sequence {
                        tunnel: [w632] -> w630
                        tunnel: w619 -> [w632]
                        frame #0 {
                          n186 = Wait (ms)(milliseconds to wait=u32 50) -> ()  [unwired: 1 out]
                        }
                      }
                      n187 = case shown="\"Velocity\"" w620 {
                        tunnel: [w635 w641 w650 w658 w676 "EP=1\r\n" ("write buffer") "Cannot perform operation.\n" ("read buffer")] -> w621
                        tunnel: w630 -> [w634 w640 w649 w663 w667 w679 w681]
                        tunnel: [w634 w640 w649 w663 w664 w679 w681] -> w629
                        tunnel: w627 -> [w636 w642 w655 _ _ _ _]
                        tunnel: w626 -> [_ _ _ w659 _ _ _]
                        tunnel: w625 -> [_ _ _ _ w668 _ _]
                        tunnel: w624 -> [_ w643 w653 _ _ _ _]
                        frame "Serial Number" {
                          n188 = Concatenate Strings("SN" ("write buffer"), "=" ("string"), w636, "\r\n" ("write buffer")) -> (w635:string)
                        }
                        frame "Temperature" {
                          n189 = Concatenate Strings("TA" ("string"), "[", w643, "]", "=" ("string"), w642, "\r\n" ("write buffer")) -> (w641:string)
                        }
                        frame "Unit Adress" {
                          n190 = Concatenate Strings("UA" ("string"), "[", w653, "]", "=" ("string"), w655, "\r\n" ("write buffer")) -> (w650:string)
                        }
                        frame "Calibration" {
                          n191 = Concatenate Strings("CC" ("string"), "=" ("string"), w659, "\r\n" ("write buffer")) -> (w658:string)
                        }
                        frame "Velocity" {
                          n192 = In Range and Coerce(upper limit=u16 18001, x=w668, lower limit=u16 0) -> (coerced(x)=w674:u32, In Range?=w672:bool)
                          n193 = Not(x=w672) -> (.not. x?=w673:bool)
                          n194 = Select(t=w674, s=w672, f=u16 0) -> (s? t:f=w666:u32)
                          n195 = Number To Decimal String(number=w666) -> (decimal integer string=w665:string)  [unwired: 1 in]
                          n196 = Concatenate Strings("VC" ("write buffer"), "=" ("string"), w665, "\r\n" ("write buffer")) -> (w676:string)
                          n197 = call "Display Message to User2"("error in (no error)"=w667, "Enable"=w673) -> ("error out"=w664:errorcluster)  [unwired: 8 in, 1 out]
                        }
                        frame "Enable Conf. EP=1" {
                        }
                        frame Default {
                        }
                      }
                      n198 = property on="read buffer" class="Str"() -> ("Value"=w617:string)  [unwired: 2 in, 2 out]
                      n199 = VISA Write(VISA resource name=w628, write buffer=w621, error in (no error)=w629) -> (error out=w631:errorcluster)  [unwired: 2 out]
                      n200 = Concatenate Strings(w617, w621) -> (w622:string)
                      n201 = property on="Serial Send" class="Bool (strict)"("Value"=FALSE ("Serial Send")) -> ()  [unwired: 2 in, 2 out]
                      n202 = flat-sequence {
                        tunnel: w631 -> [w683]
                        tunnel: [w683] -> w623
                        frame #0 {
                          n203 = Wait (ms)(milliseconds to wait=u32 50) -> ()  [unwired: 1 out]
                        }
                      }
                    }
                  }
                }
              }
              "read buffer" <- w469
              n204 = Add(x=u32 5, y=w462) -> (x+y=w461:u32)
              n205 = property on="read buffer" class="Str"(error in=w464, "Text.Scroll Position"=w461) -> (error out=w463:errorcluster)  [unwired: 1 in, 1 out]
            }
            event "Set Param.": Value Change {
              n206 = event-data() -> ()  [unwired: 1 in, 6 out]
              n207 = property on="Serial Status" class="Bool (strict)"(error in=w717) -> (error out=w716:errorcluster, "Value"=w721:bool)  [unwired: 1 in, 1 out]
              n208 = case shown="True" w721 {
                tunnel: w716 -> [w733 w746]
                tunnel: [w732 w742] -> w719
                frame False {
                  n209 = call "Display Message to User4"("error in (no error)"=w733) -> ("error out"=w732:errorcluster)  [unwired: 9 in, 1 out]
                }
                frame True {
                  w735 = FALSE ("Visible")
                  n210 = property on="Speed control" class="Bool (strict)"(error in=w746, "Visible"=FALSE) -> (error out=w745:errorcluster)  [unwired: 1 in, 1 out]
                  n211 = case shown="47" "Param to Set" {
                    tunnel: [w799 w803 w807] -> w761
                    tunnel: w745 -> [w798 w802 w806]
                    tunnel: [w798 w802 w806] -> w749
                    frame 95, Default {
                      n212 = call <vilib>:"Application Directory.vi"() -> ("Application Directory"=w801:path)
                      n213 = Build Path(base path=w801, name or relative path="data\\Marvin_EBAY_params_RRPAR000017_95_v0.2.txt") -> (appended path=w799:path)
                    }
                    frame 63 {
                      n214 = call <vilib>:"Application Directory.vi"() -> ("Application Directory"=w805:path)
                      n215 = Build Path(base path=w805, name or relative path="data\\Marvin_AHU_params_RRPAR000016_63_v0.2.txt") -> (appended path=w803:path)
                    }
                    frame 47 {
                      n216 = call <vilib>:"Application Directory.vi"() -> ("Application Directory"=w809:path)
                      n217 = Build Path(base path=w809, name or relative path="data\\Marvin_AHU_params_RRPAR000015_47_v0.2.txt") -> (appended path=w807:path)
                    }
                  }
                  n218 = property on="read buffer" class="Str"(error in=w749, "Visible"=TRUE) -> (error out=w737:errorcluster)  [unwired: 1 in, 1 out]
                  n219 = property on="CAN Data" class="Arr (strict)"(error in=w737, "Visible"=w735) -> (error out=w736:errorcluster)  [unwired: 1 in, 1 out]
                  n220 = property on="PlayPause Data Array" class="Bool (strict)"("Visible"=w735) -> ()  [unwired: 2 in, 2 out]
                  n221 = property on="Clear Data Array" class="Bool (strict)"("Visible"=w735) -> ()  [unwired: 2 in, 2 out]
                  n222 = property on="Horizontal Progress Bar" class="Slide (strict)"(error in=w736, "Visible"=TRUE, "Value"=u8 0 ("Horizontal Progress Bar")) -> (error out=w744:errorcluster)  [unwired: 1 in, 1 out]
                  n223 = call <vilib>:"Read Characters From File.vi"("file path (dialog if empty)"=w761) -> ("character string"=w762:string)  [unwired: 5 in, 3 out]
                  n224 = while {
                    shift-right: [w790] -> _
                    shift-left: w762 -> [w791]
                    shift-right: [w786] -> w747
                    shift-left: string[] [] -> [w787]
                    tunnel: w744 -> [w779]
                    tunnel: [w779] -> w759
                    stop <- w792 stop-if-true
                    n225 = Match Pattern(string=w791, regular expression="\r\n") -> (before substring=w788:string, after substring=w790:string, offset past match=w789:i32)  [unwired: 1 in, 1 out]
                    n226 = call <vilib>:"Trim Whitespace.vi"("string"=w788) -> ("trimmed string"=w785:string)  [unwired: 1 in]
                    n227 = Equal?(x=w789, y=-1) -> (x = y?=w792:bool)
                    n228 = To Upper Case(1:w785) -> (0:w783:string)
                    n229 = String Length(string=w783) -> (length=w782:i32)
                    n230 = Greater?(x=w782, y=3) -> (0:w780:bool)
                    n231 = case shown="True" w780 {
                      tunnel: w787 -> [w794 w797]
                      tunnel: [w794 w796] -> w786
                      tunnel: w783 -> [_ w795]
                      frame False {
                      }
                      frame True {
                        n232 = Build Array (concatenate)(w797, w795) -> (w796:string[])
                      }
                    }
                  }
                  n233 = property on="VISA resource name" class="VISAName"(error in=w759) -> (error out=w752:errorcluster, "Value"=w741:refnum<visa-resource-name>)  [unwired: 1 in, 1 out]
                  n234 = Build Array (concatenate)(w747, string[] ["MT", "VR", "SN"] ("array")) -> (w756:string[])
                  n235 = Array Size(array=w756) -> (size(s)=w748:i32)
                  n236 = Bundle By Name(cluster=T12 {"Minimum"=0.0, "Maximum"=0.0, "Increment"=0.0} ("Data Entry Limits"), "Minimum"=0.0, "Maximum"=w748) -> (w754:T12)
                  n237 = property on="Horizontal Progress Bar" class="Slide (strict)"(error in=w752, "Data Range"=w754) -> (error out=w740:errorcluster)  [unwired: 1 in, 1 out]
                  n238 = property on="read buffer" class="Str"(error in=w740) -> (error out=w739:errorcluster, "Text.Scroll Position"=w738:u32)  [unwired: 1 in, 1 out]
                  n239 = for {
                    tunnel: w756 -> [w770] mode=indexing
                    tunnel: w741 -> [w776]
                    tunnel: w739 -> [w775]
                    tunnel: [w767] -> w743
                    tunnel: w738 -> [w766]
                    i -> [w765]
                    n240 = Concatenate Strings(w770, "\r\n" ("string")) -> (w768:string)
                    n241 = VISA Write(VISA resource name=w776, write buffer=w768, error in (no error)=w775) -> (error out=w774:errorcluster)  [unwired: 2 out]
                    n242 = flat-sequence {
                      tunnel: w774 -> [w777]
                      tunnel: [w777] -> w767
                      frame #0 {
                        n243 = Wait (ms)(milliseconds to wait=u32 50) -> ()  [unwired: 1 out]
                      }
                    }
                    n244 = Add(x=w766, y=w765) -> (x+y=w764:u32)
                    n245 = feedback #1("") -> (w772:string)
                    n246 = Concatenate Strings(w772, w768) -> (w773:string)
                    n247 = feedback-in #1(w773) -> ()
                    n248 = property on="read buffer" class="Str"("Value"=w773, "Text.Scroll Position"=w764) -> ()  [unwired: 2 in, 2 out]
                    "Horizontal Progress Bar" <- w765
                  }
                  n249 = VISA Flush I/O Buffer(VISA resource name=w741, error in (no error)=w743) -> (error out=w742:errorcluster)  [unwired: 1 in, 1 out]
                }
              }
              n250 = property on="Serial Monitor" class="Bool (strict)"(error in=w719) -> (error out=w718:errorcluster, "Value"=w720:bool)  [unwired: 1 in, 1 out]
              n251 = case shown="False" w720 {
                tunnel: w718 -> [w730 w731]
                tunnel: [w727 w731] -> w714
                frame False {
                  w726 = TRUE ("Visible")
                  n252 = property on="PlayPause Data Array" class="Bool (strict)"("Visible"=w726) -> ()  [unwired: 2 in, 2 out]
                  n253 = property on="read buffer" class="Str"(error in=w730, "Visible"=FALSE) -> (error out=w728:errorcluster)  [unwired: 1 in, 1 out]
                  n254 = property on="Clear Data Array" class="Bool (strict)"("Visible"=w726) -> ()  [unwired: 2 in, 2 out]
                  n255 = property on="CAN Data" class="Arr (strict)"(error in=w728, "Visible"=w726) -> (error out=w727:errorcluster)  [unwired: 1 in, 1 out]
                }
                frame True {
                }
              }
              n256 = call "Display Message to User5"("error in (no error)"=w714) -> ("error out"=w713:errorcluster)  [unwired: 9 in, 1 out]
            }
            event "Help Button": Value Change {
              n257 = event-data() -> ()  [unwired: 1 in, 6 out]
              n258 = control-ref of="This VI"() -> (w818:refnum<vi>)
              n259 = property class="VI"(reference=w818, error in=w816, "FP:Transparency"=u8 25 ("Front Panel Window:Transparency")) -> (reference out=w812:refnum<vi>, error out=w815:errorcluster)
              n260 = vi-ref "Help.vi"() -> (w822:refnum<vi>)
              n261 = invoke class="VI" method="FP.Open"(reference=w822, error in=w815, "Activate"=TRUE ("Activate?"), "State"=T13."Standard") -> (error out=w821:errorcluster)  [unwired: 1 in, 4 out]
              n262 = call "Help.vi"("error in"=w821, "TesterSWVersion"="1.7") -> ("error out"=w814:errorcluster)  [unwired: 6 in]
              n263 = property class="VI"(reference=w812, error in=w814, "FP:Transparency"=u8 0 ("Front Panel Window:Transparency")) -> (error out=w813:errorcluster)  [unwired: 1 out]
            }
            event "Can Send": Value Change {
              w857 = u8 0 items=["STATUS"=128, "EXTENDED"=2, "RTR"=1, "DATA MSG"=0] ("MSGTYPE")
              w862 = u8 1 items=["Standart flag", "Extern flag"] ("Format")
              w861 = u8 0 items=["Data flag", "Remote flag"] ("Type")
              # "Send"
              n264 = event-data() -> ()  [unwired: 1 in, 6 out]
              n265 = In Range and Coerce(upper limit=u16 18001, x="Motor Speed RPM", lower limit=u16 0) -> (coerced(x)=w844:u16, In Range?=w842:bool)
              n266 = In Range and Coerce(upper limit=u16 100, x="Motor Phase Current", lower limit=u16 40) -> (coerced(x)=w833:u16, In Range?=w835:bool)
              n267 = Not(x=w842) -> (.not. x?=w843:bool)
              n268 = Not(x=w835) -> (.not. x?=w834:bool)
              n269 = call "Display Message to User"("Enable"=w843) -> ()  [unwired: 9 in, 2 out]
              n270 = Select(t=w844, s=w842, f=u16 0) -> (s? t:f=w846:u16)
              n271 = call "Display Message to User6"("Enable"=w834) -> ()  [unwired: 9 in, 2 out]
              n272 = Select(t=w833, s=w835, f=u16 0) -> (s? t:f=w828:u16)
              n273 = property on="UUT" class="DigNum (strict)"() -> ("Value"=w840:u8)  [unwired: 2 in, 2 out]
              n274 = Split Number(x=w846) -> (hi(x)=w849:u8, lo(x)=w850:u8)
              n275 = case shown="79" w840 {
                tunnel: [u32 417357607 u32 417353511 u32 417349415 u32 417345319] -> w841
                frame 95, Default {
                }
                frame 79 {
                }
                frame 63 {
                }
                frame 47 {
                }
              }
              n276 = case shown="79" w840 {
                tunnel: [w881 w890 w903 w917] -> w855
                tunnel: w850 -> [w880 w889 w902 w916]
                tunnel: w849 -> [w879 w888 w901 w915]
                tunnel: "Motor Speed RPM" -> [w876 w885 _ _]
                tunnel: "Speed control" -> [_ _ w894 w908]
                tunnel: "Motor Over Temp" -> [_ _ w893 w907]
                tunnel: w828 -> [_ _ _ w904]
                frame 47, Default {
                  w878 = u8 0 ("element")
                  n277 = case shown="1, Default" w876 {
                    tunnel: [u8 1 ("element") u8 0 ("element")] -> w875
                    frame 1, Default {
                    }
                    frame 0 {
                    }
                  }
                  n278 = Build Array(u8 1 ("element"), w880, w879, w875, w878, w878, w878, w878) -> (w881:u8[])
                }
                frame 63 {
                  w886 = u8 0 ("element")
                  n279 = case shown="1, Default" w885 {
                    tunnel: [u8 1 ("element") u8 0 ("element")] -> w884
                    frame 1, Default {
                    }
                    frame 0 {
                    }
                  }
                  n280 = Build Array(u8 1 ("element"), w889, w888, w884, w886, w886, w886, w886) -> (w890:u8[])
                }
                frame 95 {
                  w899 = u8 0 ("element")
                  n281 = Boolean To (0,1)(Boolean=w894) -> (0, 1=w897:i16)
                  n282 = Boolean To (0,1)(Boolean=w893) -> (0, 1=w898:i16)
                  n283 = To Unsigned Byte Integer(number=w897) -> (unsigned 8bit integer=w896:u8)
                  n284 = To Unsigned Byte Integer(number=w898) -> (unsigned 8bit integer=w895:u8)
                  n285 = Build Array(u8 1 ("element"), w902, w901, w896, w895, w899, w899, w899) -> (w903:u8[])
                }
                frame 79 {
                  n286 = Split Number(x=w904) -> (hi(x)=w905:u8, lo(x)=w906:u8)
                  n287 = Boolean To (0,1)(Boolean=w908) -> (0, 1=w911:i16)
                  n288 = Boolean To (0,1)(Boolean=w907) -> (0, 1=w912:i16)
                  n289 = To Unsigned Byte Integer(number=w911) -> (unsigned 8bit integer=w910:u8)
                  n290 = To Unsigned Byte Integer(number=w912) -> (unsigned 8bit integer=w909:u8)
                  n291 = Build Array(u8 1 ("element"), w916, w915, w910, w909, w906, w905, u8 0 ("element")) -> (w917:u8[])
                }
              }
              n292 = Array Size(array=w855) -> (size(s)=w860:i32)
              n293 = call "Array Data to Single Num in Hex.vi"("aDATA"=w855) -> ("Numeric"=→"Data Send":u64)  [unwired: 10 in]
              n294 = To Unsigned Byte Integer(number=w860) -> (unsigned 8bit integer=w858:u8)
              n295 = call "CANAnalData.vi"("ID"=w841, "Data"=w855, "Config"=w853) -> ()  [unwired: 4 in, 5 out]
              n296 = Bundle By Name(cluster=T10 {"ID"=0, "MSGTYPE"=0, "LEN"=0, "aDATA"=[]} ("MsgTX 2"), "ID"=w841, "MSGTYPE"=w857, "LEN"=w858, "aDATA"=w855) -> (w856:T10)
              n297 = Unbundle By Name(w856) -> ("ID"=w870:u32, "LEN"=w871:u8, "aDATA"=w872:u8[])  [unwired: 1 out]
              n298 = property class="Clust (strict)"(reference=w853) -> ("Value"=w869:T8)  [unwired: 1 in, 2 out]
              n299 = Bundle By Name(cluster=T14 {"ID"=0, "TimeStamp"=0, "TimeFlag"=0, "SendType"=0, "RemoteFlag"=0, "ExternFlag"=0, "DataLen"=0, "Data"=[], "Reserved"=[]} ("Send"), "ID"=w870, "RemoteFlag"=w861, "ExternFlag"=w862, "DataLen"=w871, "Data"=w872) -> (w867:T14)
              n300 = Unbundle By Name(w869) -> ("DevType"=w863:T2, "DevIndex"=w864:u32, "CanIndex"=w865:T3)
              n301 = Build Array(w867) -> (w866:T14[])
              n302 = call "VCI_Transmit.vi"("Buffer"=w866, "CANIndex"=w865, "DevIndex"=w864, "DevType"=w863) -> ()  [unwired: 1 in, 7 out]
            }
            event "Graph Button": Value Change {
              w922 = FALSE ("Visible")
              n303 = event-data() -> ()  [unwired: 1 in, 6 out]
              n304 = Not(x="Graph Button") -> (.not. x?=w923:bool)
              n305 = property on="PlayPause Data Array" class="Bool (strict)"("Visible"=w923) -> ()  [unwired: 2 in, 2 out]
              n306 = property on="CAN Data" class="Arr (strict)"(error in=w924, "Visible"=w923) -> (error out=w925:errorcluster)  [unwired: 1 in, 1 out]
              n307 = property on="Clear Data Array" class="Bool (strict)"("Visible"=w923) -> ()  [unwired: 2 in, 2 out]
              n308 = property on="Waveform Chart" class="WFChart (strict)"(error in=w925, "Visible"="Graph Button") -> (error out=w927:errorcluster)  [unwired: 1 in, 1 out]
              n309 = property on="Serial Monitor" class="Bool (strict)"(error in=w927) -> (error out=w941:errorcluster, "Value"=w942:bool)  [unwired: 1 in, 1 out]
              n310 = case shown="True" w942 {
                tunnel: w941 -> [w949 w954]
                tunnel: [w947 w951] -> w930
                frame False {
                  n311 = property on="read buffer" class="Str"(error in=w949, "Visible"=FALSE) -> (error out=w947:errorcluster)  [unwired: 1 in, 1 out]
                }
                frame True {
                  w950 = FALSE ("Visible")
                  n312 = property on="PlayPause Data Array" class="Bool (strict)"("Visible"=w950) -> ()  [unwired: 2 in, 2 out]
                  n313 = property on="read buffer" class="Str"(error in=w954, "Visible"=TRUE) -> (error out=w952:errorcluster)  [unwired: 1 in, 1 out]
                  n314 = property on="Clear Data Array" class="Bool (strict)"("Visible"=w950) -> ()  [unwired: 2 in, 2 out]
                  n315 = property on="CAN Data" class="Arr (strict)"(error in=w952, "Visible"=w950) -> (error out=w951:errorcluster)  [unwired: 1 in, 1 out]
                }
              }
              n316 = property on="Serial Monitor" class="Bool (strict)"(error in=w930, "Value"=FALSE ("Serial Monitor")) -> (error out=w928:errorcluster)  [unwired: 1 in, 1 out]
              n317 = property on="Index" class="Ring (strict)"(error in=w928, "Visible"=w922) -> (error out=w938:errorcluster)  [unwired: 1 in, 1 out]
              n318 = property on="Value 1/2" class="Enum (strict)"(error in=w938, "Visible"=w922) -> (error out=w937:errorcluster)  [unwired: 1 in, 1 out]
              n319 = property on="Value" class="DigNum (strict)"(error in=w937, "Visible"=w922) -> (error out=w936:errorcluster)  [unwired: 1 in, 1 out]
              n320 = property on="SetGet" class="Enum (strict)"(error in=w936, "Visible"=w922) -> (error out=w935:errorcluster)  [unwired: 1 in, 1 out]
              n321 = property on="Serial Send" class="Bool (strict)"(error in=w935, "Visible"=w922) -> (error out=w933:errorcluster)  [unwired: 1 in, 1 out]
              n322 = property on="Clear Monitor" class="Bool"(error in=w933, "Visible"=w922) -> (error out=w932:errorcluster)  [unwired: 1 in, 1 out]
              n323 = property on="Function" class="Enum (strict)"(error in=w932, "Visible"=w922) -> (error out=w934:errorcluster)  [unwired: 1 in, 1 out]
              n324 = property on="Index" class="Ring (strict)"(error in=w934, "Visible"=w922) -> (error out=w939:errorcluster)  [unwired: 1 in, 1 out]
              n325 = property on="read buffer" class="Str"(error in=w939, "Visible"=w922) -> (error out=w931:errorcluster)  [unwired: 1 in, 1 out]
            }
            event "Serial Com": Value Change {
              n326 = event-data() -> ()  [unwired: 1 in, 6 out]
              n327 = property on="Serial Com" class="Bool"(error in=w959, "Visible"=FALSE) -> (error out=w958:errorcluster)  [unwired: 1 in, 1 out]
              n328 = property on="VISA resource name" class="VISAName"(error in=w958, "Visible"=TRUE) -> (error out=w956:errorcluster)  [unwired: 1 in, 1 out]
            }
            event "VISA resource name": Value Change {
              n329 = event-data() -> ()  [unwired: 1 in, 1 out]
              n330 = control-ref of="This VI"() -> (w965:refnum<vi>)
              n331 = call "Serial InitMarvin.vi"("error in (no error)"=w974, "VI reference (current VI)"=w965, "VISA Refnum in"="VISA resource name") -> ("error out"=w983:errorcluster, "Boolean"=w971:bool)  [unwired: 7 in]
              n332 = property on="Serial Status" class="Bool (strict)"(error in=w983, "Value"=w971) -> (error out=w977:errorcluster)  [unwired: 1 in, 1 out]
              n333 = property on="VISA resource name" class="VISAName"(error in=w977, "Visible"=FALSE) -> (error out=w976:errorcluster)  [unwired: 1 in, 1 out]
              n334 = property on="Serial Com" class="Bool"(error in=w976, "Visible"=TRUE) -> (error out=w969:errorcluster)  [unwired: 1 in, 1 out]
              n335 = call "Serial.vi"("error in (no error)"=w969, "Clear Log"=TRUE, "VISA resource name"="VISA resource name") -> ("error out"=w967:errorcluster)  [unwired: 7 in, 1 out]
              n336 = call <vilib>:"Clear Errors.vi"("error in (no error)"=w967) -> ("error out"=w973:errorcluster)  [unwired: 5 in, 1 out]
              n337 = case shown="True" w971 {
                tunnel: w973 -> [w984 w987]
                tunnel: [w984 w986] -> w972
                tunnel: "VISA resource name" -> [_ w985]
                frame False {
                }
                frame True {
                  n338 = VISA Flush I/O Buffer(VISA resource name=w985, error in (no error)=w987) -> (error out=w986:errorcluster)  [unwired: 1 in, 1 out]
                }
              }
            }
            event "Stop": Value Change {
              n339 = event-data() -> ()  [unwired: 1 in, 6 out]
              n340 = Flush Queue(queue=w993, error in (no error)=w992) -> (queue out=w991:refnum<queue>, error out=w990:errorcluster)  [unwired: 1 out]
              n341 = Release Queue(queue=w991, error in (no error)=w990) -> (error out=w989:errorcluster)  [unwired: 1 in, 2 out]
            }
            event "Refresh Button": Value Change {
              n342 = event-data() -> ()  [unwired: 1 in, 6 out]
              n343 = Release Queue(queue=w999, error in (no error)=w1000) -> (error out=w998:errorcluster)  [unwired: 1 in, 2 out]
            }
          }
          n344 = Unbundle By Name(w280) -> ("status"=w286:bool)
          n345 = Or(x=w286, y=w278) -> (x .or. y?=w285:bool)
        }
        n346 = while {
          shift-right: [w120] -> _
          shift-left: w98 -> [w122]
          shift-right: [w118] -> _
          shift-left: _ -> [w119]
          shift-right: [w114] -> _
          shift-left: w97 -> [w114]
          shift-right: [w104] -> w93
          shift-left: w94 -> [w113]
          shift-right: [w106] -> _
          shift-left: cluster{"Frame Data":u64, "Frame ID":u32}[] [] ("Array 3") -> [w108]
          stop <- w121 stop-if-true
          n347 = Dequeue Element(queue=w122, error in (no error)=w114) -> (queue out=w120:refnum<queue>, element=w115:T9, error out=w121:errorcluster)  [unwired: 1 in, 1 out]
          n348 = for {
            tunnel: [w264] -> w117 mode=indexing
            tunnel: w115 -> [w266] mode=indexing
            tunnel: [w265] -> w116 mode=indexing
            tunnel: [w263] -> w112 mode=indexing
            tunnel: [w262] -> w111 mode=indexing
            shift-right: [w262] -> _
            shift-left: _ -> [w261]
            n349 = Unbundle By Name(w266) -> ("ID"=w263:u32, "aDATA"=w265:u8[])
            n350 = call "Array Data to Single Num in Hex.vi"("aDATA"=w265) -> ("Numeric"=w264:u64)  [unwired: 10 in]
            n351 = case shown="Default" w263 {
              tunnel: w264 -> [_ w271]
              tunnel: w263 -> [_ w270]
              tunnel: [w267 w269] -> w262
              tunnel: w261 -> [w267 _]
              frame 0 {
              }
              frame Default {
                n352 = Bundle By Name(cluster=cluster{"Frame Data":u64, "Frame ID":u32} {"Frame Data"=0, "Frame ID"=0} ("Cluster"), "Frame ID"=w270, "Frame Data"=w271) -> (w269:cluster{"Frame Data":u64, "Frame ID":u32})
              }
            }
          }
          n353 = case shown="True" "PlayPause Data Array" {
            tunnel: w111 -> [w125 _]
            tunnel: w108 -> [w124 w126]
            tunnel: [w123 w126] -> w107
            frame False {
              n354 = Build Array (concatenate)(w125, w124) -> (w123:cluster{"Frame Data":u64, "Frame ID":u32}[])
            }
            frame True {
            }
          }
          n355 = Build Array (concatenate)(w117, w119) -> (w118:u64[][])
          "Array" <- w118
          n356 = Select(t=cluster{"Frame Data":u64, "Frame ID":u32}[] [], s="Clear Data Array", f=w107) -> (s? t:f=w106:cluster{"Frame Data":u64, "Frame ID":u32}[])
          "CAN Data" <- w106
          n357 = for {
            tunnel: w116 -> [w130] mode=indexing
            tunnel: w112 -> [w128] mode=indexing
            shift-right: [w127] -> w104
            shift-left: w113 -> [w129]
            n358 = case shown="417474367, 417474383, 417474399" w128 {
              tunnel: w130 -> [_ w160 w198 w256]
              tunnel: [w131 w132 w189 w228] -> w127
              tunnel: w129 -> [w131 w137 w189 w229]
              frame Default {
              }
              frame 417408831, 417408847, 417408863 {
                # "Frame ID\n0x18E1273F"
                n359 = Index Array(array=w160, index #1=0 ("index"), index #2=1 ("index"), index #3=2 ("index"), index #4=3 ("index"), index #5=4 ("index"), index #6=5 ("index"), index #7=6 ("index"), index #8=7 ("index")) -> (element #1=w144:u8, element #2=w146:u8, element #3=w147:u8, element #4=w151:u8, element #5=w154:u8, element #6=w158:u8, element #7=w159:u8, element #8=w157:u8)
                n360 = Join Numbers(hi=w159, lo=w158) -> ((hi.lo)=w178:u16)
                n361 = Join Numbers(hi=w147, lo=w146) -> ((hi.lo)=w148:u16)
                n362 = Number To Hexadecimal String(2:w178) -> (0:w177:string)  [unwired: 1 in]
                n363 = Number To Hexadecimal String(2:w157) -> (0:w171:string)  [unwired: 1 in]
                n364 = Number To Hexadecimal String(2:w144) -> (0:w145:string)  [unwired: 1 in]
                n365 = Number To Hexadecimal String(2:w148) -> (0:w149:string)  [unwired: 1 in]
                n366 = Number To Hexadecimal String(2:w151) -> (0:w152:string)  [unwired: 1 in]
                n367 = Number To Hexadecimal String(2:w154) -> (0:w155:string)  [unwired: 1 in]
                n368 = Hexadecimal String To Number(string=w145) -> (number=w142:u32)  [unwired: 2 in, 1 out]
                n369 = Hexadecimal String To Number(string=w149) -> (number=w150:u32)  [unwired: 2 in, 1 out]
                n370 = Hexadecimal String To Number(string=w152) -> (number=w153:u32)  [unwired: 2 in, 1 out]
                n371 = Hexadecimal String To Number(string=w155) -> (number=w156:u32)  [unwired: 2 in, 1 out]
                n372 = Hexadecimal String To Number(string=w171) -> (number=w170:u32)  [unwired: 2 in, 1 out]
                n373 = Hexadecimal String To Number(string=w177) -> (number=w176:u32)  [unwired: 2 in, 1 out]
                n374 = To Unsigned Word Integer(number=w142) -> (unsigned 16bit integer=→"ECS State":u16)
                n375 = To Double Precision Float(number=w150) -> (double precision float=w135:dbl)
                "Motor Speed RPM" <- w135
                n376 = To Double Precision Float(number=w176) -> (double precision float=w173:dbl)
                n377 = To Double Precision Float(number=w170) -> (double precision float=→"DC Current":dbl)
                n378 = To Double Precision Float(number=w153) -> (double precision float=w141:dbl)
                n379 = To Double Precision Float(number=w156) -> (double precision float=w139:dbl)
                n380 = To Double Precision Float(number=u32 10 ("y")) -> (double precision float=w174:dbl)
                n381 = Subtract(x=w139, y=50.0 ("x")) -> (x-y=→"Power transistor Heat sink Temp.":dbl)
                n382 = Subtract(x=w141, y=50.0 ("x")) -> (x-y=→"Motor Stator Temp.":dbl)
                n383 = Divide(x=w173, y=w174) -> (x/y=→"DC Voltage":dbl)
                n384 = case shown="True" FALSE {
                  tunnel: w137 -> [w179 w182]
                  tunnel: [w179 w181] -> w132
                  tunnel: w135 -> [_ w180]
                  frame False {
                  }
                  frame True {
                    n385 = disable-structure shown="Disabled" {
                      disable-tunnel: w180 -> [w186 _]
                      frame Disabled {
                        n386 = call <vilib>:"Application Directory.vi"() -> ("Application Directory"=w184:path)
                        n387 = Build Path(base path=w184, name or relative path="RPM Log.lvm") -> (appended path=w185:path)
                        n388 = call "Write To Measurement File"("Signals"=w186, "Filename"=w185) -> ()  [unwired: 15 in, 3 out]
                      }
                      frame Enabled {
                      }
                    }
                    n389 = Build Array (concatenate)(w180, w182) -> (w181:dbl[])
                  }
                }
              }
              frame 417539903, 417539919, 417539935 {
                # "Framde ID\n0x18E3273F"
                n390 = property on="UUT" class="DigNum (strict)"() -> ("Value"=w188:u8)  [unwired: 2 in, 2 out]
                n391 = Index Array(array=w198, index #1=0 ("index"), index #2=1 ("index")) -> (element #1=w196:u8, element #2=w191:u8)
                n392 = case shown="Default" w188 {
                  tunnel: [0 1 2] -> w187
                  frame Default {
                  }
                  frame 95 {
                  }
                  frame 79 {
                  }
                }
                n393 = Number To Boolean Array(number=w196) -> (Boolean array=w195:bool[])
                n394 = Number To Boolean Array(number=w191) -> (Boolean array=w193:bool[])
                n395 = Boolean To (0,1)(Boolean=w193) -> (0, 1=w190:i16[])
                n396 = Boolean To (0,1)(Boolean=w195) -> (0, 1=w194:i16[])
                n397 = case shown="79, 95" w188 {
                  tunnel: w190 -> [_ w203]
                  tunnel: w187 -> [_ w202]
                  frame 0, Default {
                  }
                  frame 79, 95 {
                    n398 = for {
                      tunnel: w203 -> [w208] mode=indexing
                      tunnel: w202 -> [w204]
                      i -> [w205]
                      stop <- w206 stop-if-true
                      n399 = Not Equal To 0?(x=w208) -> (x != 0?=w207:bool)
                      n400 = case shown="2" w205 {
                        tunnel: w207 -> [w209 w210 w211]
                        frame 0, Default {
                          "Ambient Sensor temp" <- w209
                        }
                        frame 1 {
                          "Ambient Over temp" <- w210
                        }
                        frame 2 {
                          "Hall Sensor Fault" <- w211
                        }
                      }
                      n401 = Equal?(x=w205, y=w204) -> (x = y?=w206:bool)
                    }
                  }
                }
                n402 = for {
                  tunnel: w194 -> [w213] mode=indexing
                  i -> [w214]
                  n403 = Not Equal To 0?(x=w213) -> (x != 0?=w212:bool)
                  n404 = case shown="0, Default" w214 {
                    tunnel: w212 -> [w215 w216 w217 w218 w219 w220 w221 w222]
                    frame 0, Default {
                      "Drive Sensor temp Failure" <- w215
                    }
                    frame 1 {
                      "Drive Over temperature" <- w216
                    }
                    frame 2 {
                      "Motor Sensor temp Fauilre" <- w217
                    }
                    frame 3 {
                      "Motor Over temperature" <- w218
                    }
                    frame 4 {
                      "Derated drive temp" <- w219
                    }
                    frame 5 {
                      "Under voltage/Over voltage" <- w220
                    }
                    frame 6 {
                      "Commutation err" <- w221
                    }
                    frame 7 {
                      "Speed error" <- w222
                    }
                  }
                }
              }
              frame 417474367, 417474383, 417474399 {
                w239 = "."
                # "Frame ID\n0x18E2273F"
                n405 = Index Array(array=w256, index #1=0 ("index")) -> (element #1=w254:u8, element #2=w252:u8, element #3=w233:u8, element #4=w234:u8, element #5=w235:u8, element #6=w236:u8)  [unwired: 5 in]
                n406 = Split Number(x=w235) -> (hi(x)=w247:u8, lo(x)=w246:u8)
                n407 = Split Number(x=w236) -> (hi(x)=w245:u8, lo(x)=w244:u8)
                n408 = Join Numbers(hi=w234, lo=w233) -> ((hi.lo)=w224:u16)
                n409 = Number To Hexadecimal String(2:w224) -> (0:w225:string)  [unwired: 1 in]
                n410 = Number To Decimal String(number=w247) -> (decimal integer string=w243:string)  [unwired: 1 in]
                n411 = Number To Decimal String(number=w246) -> (decimal integer string=w242:string)  [unwired: 1 in]
                n412 = Number To Decimal String(number=w245) -> (decimal integer string=w241:string)  [unwired: 1 in]
                n413 = Number To Decimal String(number=w244) -> (decimal integer string=w240:string)  [unwired: 1 in]
                n414 = Hexadecimal String To Number(string=w225) -> (number=w226:u32)  [unwired: 2 in, 1 out]
                n415 = To Double Precision Float(number=w226) -> (double precision float=w223:dbl)
                n416 = Number To Hexadecimal String(2:w252) -> (0:w250:string)  [unwired: 1 in]
                n417 = To Double Precision Float(number=w254) -> (double precision float=→"Motor Phase Current RMS":dbl)
                n418 = Multiply(x=w223, y=u16 1) -> (x*y=w231:dbl)
                n419 = Concatenate Strings(w243, w239, w242, w239, w241, w239, w240) -> (→"Driver Version":string)
                n420 = To Double Precision Float(number=w231) -> (double precision float=w230:dbl)
                "Motor Phase Current" <- w230
                n421 = Hexadecimal String To Number(string=w250) -> (number=w251:u32)  [unwired: 2 in, 1 out]
                n422 = To Double Precision Float(number=w251) -> (double precision float=w249:dbl)
                n423 = Subtract(x=w249, y=50.0) -> (x-y=→"Ambient Temperature":dbl)
                n424 = case shown="True" TRUE {
                  tunnel: w229 -> [w257 w260]
                  tunnel: [w257 w259] -> w228
                  tunnel: w230 -> [_ w258]
                  frame False {
                  }
                  frame True {
                    n425 = Build Array (concatenate)(w258, w260) -> (w259:dbl[])
                  }
                }
              }
            }
            "Waveform Chart" <- w127
            "Array 2" <- w127
          }
        }
      }
      frame "Stop" {
        n426 = Release Queue(queue=w1008, error in (no error)=w1010) -> (error out=w1009:errorcluster)  [unwired: 1 in, 2 out]
        n427 = flat-sequence {
          tunnel: w1007 -> [w1011]
          tunnel: [TRUE ("Stop")] -> w1006
          frame #0 {
            w1017 = u8[] [1, 0, 0, 0, 0, 0, 0, 0] ("Data 2")
            w1019 = u8 0 items=["STATUS"=128, "EXTENDED"=2, "RTR"=1, "DATA MSG"=0] ("MSGTYPE")
            w1024 = u8 1 items=["Standart flag", "Extern flag"] ("Format")
            w1023 = u8 0 items=["Data flag", "Remote flag"] ("Type")
            n428 = property on="Serial Status" class="Bool (strict)"() -> ("Value"=w1012:bool)  [unwired: 2 in, 2 out]
            n429 = property on="UUT" class="DigNum (strict)"() -> ("Value"=w1014:u8)  [unwired: 2 in, 2 out]
            n430 = case shown="True" w1012 {
              frame False {
              }
              frame True {
                n431 = property on="VISA resource name" class="VISAName"() -> ("Value"=w1035:refnum<visa-resource-name>)  [unwired: 2 in, 2 out]
                n432 = VISA Close(VISA resource name=w1035) -> ()  [unwired: 1 in, 1 out]
              }
            }
            n433 = case shown="95, Default" w1014 {
              tunnel: [u32 417357607 u32 417349415 u32 417345319] -> w1013
              frame 95, Default {
              }
              frame 63 {
              }
              frame 47 {
              }
            }
            n434 = property on="Graph Button" class="Bool (strict)"("Value"=FALSE ("Graph Button")) -> ()  [unwired: 2 in, 2 out]
            n435 = Array Size(array=w1017) -> (size(s)=w1022:i32)
            n436 = To Unsigned Byte Integer(number=w1022) -> (unsigned 8bit integer=w1020:u8)
            n437 = Bundle By Name(cluster=T10 {"ID"=0, "MSGTYPE"=0, "LEN"=0, "aDATA"=[]} ("MsgTX 2"), "ID"=w1013, "MSGTYPE"=w1019, "LEN"=w1020, "aDATA"=w1017) -> (w1018:T10)
            n438 = call "CANAnalData.vi"("ID"=w1013, "Data"=w1017, "Config"=w1011) -> ()  [unwired: 4 in, 5 out]
            n439 = call "Array Data to Single Num in Hex.vi"("aDATA"=w1017) -> ("Numeric"=w1016:u64)  [unwired: 10 in]
            n440 = property on="Data Send" class="DigNum (strict)"("Value"=w1016) -> ()  [unwired: 2 in, 2 out]
            n441 = Unbundle By Name(w1018) -> ("ID"=w1032:u32, "LEN"=w1033:u8, "aDATA"=w1034:u8[])  [unwired: 1 out]
            n442 = property class="Clust (strict)"(reference=w1011) -> ("Value"=w1031:T8)  [unwired: 1 in, 2 out]
            n443 = Bundle By Name(cluster=T14 {"ID"=0, "TimeStamp"=0, "TimeFlag"=0, "SendType"=0, "RemoteFlag"=0, "ExternFlag"=0, "DataLen"=0, "Data"=[], "Reserved"=[]} ("Send"), "ID"=w1032, "RemoteFlag"=w1023, "ExternFlag"=w1024, "DataLen"=w1033, "Data"=w1034) -> (w1029:T14)
            n444 = Unbundle By Name(w1031) -> ("DevType"=w1025:T2, "DevIndex"=w1026:u32, "CanIndex"=w1027:T3)
            n445 = Build Array(w1029) -> (w1028:T14[])
            n446 = call "VCI_Transmit.vi"("Buffer"=w1028, "CANIndex"=w1027, "DevIndex"=w1026, "DevType"=w1025) -> ()  [unwired: 1 in, 7 out]
          }
          frame #1 {
          }
        }
      }
    }
  }
  n447 = disable-structure shown="Disabled" {
    frame Disabled {
      n448 = control-ref of="Config_CANAT"() -> ()  [unwired: 1 out]
      n449 = control-ref of="UUT"() -> ()  [unwired: 1 out]
    }
    frame Enabled {
    }
  }
